vi "220117-VNA RP FLAT.vi"() -> ()   [LabVIEW 2021]
uses:
  b7fd31b3-4c8f-4ae8-a038-7c142e2eb182.vi
  <vilib>/Analysis/baseanly.llb/Mean (DBL).vi
  <vilib>/Utility/file.llb/Write Delimited Spreadsheet (DBL).vi
  <vilib>/Comparison/Equal/Equal Functor/Equal Functor.lvclass
  <vilib>/Analysis/NI_AALBase.lvlib
panel:
  in  "BTN CONNECT":bool
  in  "RP VNA SETTING":T1={"F start"=200000, "F stop"=2000500, "Sweep size"=1000, "Decimation"=5000, "F_corr"=0, "Ph_OUT1"=0, "Ph_OUT2"=0, "OUT_Lvl1"=32700, "OUT_Lvl2"=32700, "GPIO"=0}
  in  "Amplitude(1V)":dbl=0.3 format="%#_13g"
  out "RP CONNECT":bool
  in  "VOA Calibration cluster":cluster{"PUMP":dbl[], "PROBE":dbl[]}
  out "TRACK DATA REL NO SMOOTHING":dbl[][](array[numeric])
  out "TRACK DATA ABS NO SMOOTHING":dbl[][](array[numeric])
  in  "BTN SAVE TRACK":bool
  in  "BTN STOP TRACK":bool
  out "TRACK REPOSITERY":path
  out "TRACK DATA REL":dbl[][](array[numeric])
  out "TRACK DATA ABS":dbl[][](array[numeric])
  out "Track File List":path[](array[path])
  out "Track Repositery List":path[](array[path])
  out "CHANNEL CHOSEN":i32
  in  "TRACK-STOP":bool
  out "STATUS":string="STOP"
  out "track data":dbl[](array[numeric])=[495490.5081042979, 495481.56129759253, 495478.2328599854, 495479.84884744807, 495476.377462383, 495478.7819904735]
  out "Information tips":string
  in  "PANEL VNA":bool
  in  "PANEL TRACKING":bool
  in  "BTN STOP":bool
  in  "PANEL GENERAL SETTINGS":bool
  in  "PANEL TRACK SETTINGS":bool
  out "MAIN TAB":T2(tab)
  out "ACQ Indicator":bool
  in  "PUMP":dbl(slide)=100.0 min=0.0 max=100.0 step=0.1 scale=0.0..100.0
  in  "PROBE":dbl(slide)=100.0 min=0.0 max=100.0 step=0.1 scale=0.0..100.0
  in  "BTN RESET VNA":bool
  in  "SPAN":dbl=1900.0 format="%#5.1f"
  in  "STOP":dbl=2000.0 format="%#5.1f"
  in  "CENTER":dbl=1050.0 format="%#5.1f"
  in  "BTN SAVE VNA STG TO TRACK":bool
  in  "BTN AF VNA":bool
  out "MAGNITUDE/PHASE":cluster{cluster{dbl, dbl}[]}[](graph)
  in  "CHANNEL CHOICE VNA":T3(radio)
  in  "BTN Center to max":bool
  in  "BTN ZOOM-":bool
  in  "BTN ZOOM+":bool
  in  "START":dbl=200.0 format="%#5.1f"
  out "SPACING":dbl=1900.0 min=0.0 max=100.0 step=0.5 format="%#5.1f"
  in  "Points N°":i32=1000 min=600 max=5000 step=1 format="%#4.4g"
  in  "BTN LOOP VNA":bool
  in  "BTN RUN VNA":bool
  in  "Hide/Show track data channel":bool[](array[boolean])
  in  "BTN AUTOSAVE RAW DATA":bool=TRUE
  in  "COMMENTS":string
  in  "ASSAY NAME":string
  in  "DELAY AFTER SWITCH (s)":i32
  in  "N°POINTS TO DISPLAY":i32=200
  in  "DISPLAY OPTION":u16(ring) items=["Absolute frequency", "Relative frequency (ppm)"]
  in  "DELAY BETWEEN TRIG (s)":i32
  in  "AVERAGE/POINT":dbl=1.0
  out "LIVE TRACK":dbl[][](graph)
  out "CHANNELS IND TRACK":T3(radio)
  in  "BTN RUN TRACK":bool
  in  "TEMPORAL SMOOTHING":i32=15
  in  "BTN NEW TRACK":bool
  in  "BTN PAUSE TRACK":bool
  in  "CHANNELS PARAMETERS":T4(array[cluster])=[{"START 2"=200.0, "STOP 2"=2000.5, "CENTER 2"=1050.0, "SPAN 2"=1800.0, "CHANNEL TRACK ?"=FALSE, "PUMP"=100.0, "PROBE"=100.0, "Points N° 2"=1000, "SPACING 2"=100.0}, {"START 2"=200.0, "STOP 2"=2000.0, "CENTER 2"=1100.0, "SPAN 2"=1800.0, "CHANNEL TRACK ?"=FALSE, "PUMP"=100.0, "PROBE"=100.0, "Points N° 2"=1000, "SPACING 2"=1800.0}, {"START 2"=200.0, "STOP 2"=2000.0, "CENTER 2"=1100.0, "SPAN 2"=1800.0, "CHANNEL TRACK ?"=FALSE, "PUMP"=100.0, "PROBE"=100.0, "Points N° 2"=1000, "SPACING 2"=1800.0}, {"START 2"=200.0, "STOP 2"=2000.0, "CENTER 2"=1100.0, "SPAN 2"=1800.0, "CHANNEL TRACK ?"=FALSE, "PUMP"=100.0, "PROBE"=100.0, "Points N° 2"=1000, "SPACING 2"=1800.0}, {"START 2"=200.0, "STOP 2"=2000.0, "CENTER 2"=1100.0, "SPAN 2"=1800.0, "CHANNEL TRACK ?"=FALSE, "PUMP"=100.0, "PROBE"=100.0, "Points N° 2"=1000, "SPACING 2"=1800.0}, {"START 2"=200.0, "STOP 2"=2000.0, "CENTER 2"=1100.0, "SPAN 2"=1800.0, "CHANNEL TRACK ?"=FALSE, "PUMP"=100.0, "PROBE"=100.0, "Points N° 2"=1000, "SPACING 2"=1800.0}, {"START 2"=200.0, "STOP 2"=2000.0, "CENTER 2"=1100.0, "SPAN 2"=1800.0, "CHANNEL TRACK ?"=FALSE, "PUMP"=100.0, "PROBE"=100.0, "Points N° 2"=1000, "SPACING 2"=1800.0}, {"START 2"=200.0, "STOP 2"=2000.0, "CENTER 2"=1100.0, "SPAN 2"=1800.0, "CHANNEL TRACK ?"=FALSE, "PUMP"=100.0, "PROBE"=100.0, "Points N° 2"=1000, "SPACING 2"=1800.0}, {"START 2"=200.0, "STOP 2"=2000.0, "CENTER 2"=1100.0, "SPAN 2"=1800.0, "CHANNEL TRACK ?"=FALSE, "PUMP"=100.0, "PROBE"=100.0, "Points N° 2"=1000, "SPACING 2"=1800.0}, {"START 2"=200.0, "STOP 2"=2000.0, "CENTER 2"=1100.0, "SPAN 2"=1800.0, "CHANNEL TRACK ?"=FALSE, "PUMP"=100.0, "PROBE"=100.0, "Points N° 2"=1000, "SPACING 2"=1800.0}, {"START 2"=200.0, "STOP 2"=2000.0, "CENTER 2"=1100.0, "SPAN 2"=1800.0, "CHANNEL TRACK ?"=FALSE, "PUMP"=100.0, "PROBE"=100.0, "Points N° 2"=1000, "SPACING 2"=1800.0}, {"START 2"=200.0, "STOP 2"=2000.0, "CENTER 2"=1100.0, "SPAN 2"=1800.0, "CHANNEL TRACK ?"=FALSE, "PUMP"=100.0, "PROBE"=100.0, "Points N° 2"=1000, "SPACING 2"=1800.0}, {"START 2"=200.0, "STOP 2"=2000.0, "CENTER 2"=1100.0, "SPAN 2"=1800.0, "CHANNEL TRACK ?"=FALSE, "PUMP"=100.0, "PROBE"=100.0, "Points N° 2"=1000, "SPACING 2"=1800.0}, {"START 2"=200.0, "STOP 2"=2000.0, "CENTER 2"=1100.0, "SPAN 2"=1800.0, "CHANNEL TRACK ?"=FALSE, "PUMP"=100.0, "PROBE"=100.0, "Points N° 2"=1000, "SPACING 2"=1800.0}, {"START 2"=200.0, "STOP 2"=2000.0, "CENTER 2"=1100.0, "SPAN 2"=1800.0, "CHANNEL TRACK ?"=FALSE, "PUMP"=100.0, "PROBE"=100.0, "Points N° 2"=1000, "SPACING 2"=1800.0}, {"START 2"=200.0, "STOP 2"=2000.0, "CENTER 2"=1100.0, "SPAN 2"=1800.0, "CHANNEL TRACK ?"=FALSE, "PUMP"=100.0, "PROBE"=100.0, "Points N° 2"=1000, "SPACING 2"=1800.0}] {"SPACING 2" min=0.0 max=100.0 step=0.5; "Points N° 2" min=0 max=100 step=1; "PROBE" min=0.0 max=100.0 step=0.5; "PUMP" min=0.0 max=100.0 step=0.5}
  out "CHANNEL IND SETTINGS":T5(radio)
  in  "TRACK DATA PARAMETERS":cluster{"MAIN FOLDER":path}={"MAIN FOLDER"=path "C:/SensWay Data"}
  in  "SPECTRUM POST PROCESSING PARAMETERS":cluster{"N° SMOOTHING POINTS":i32}={"N° SMOOTHING POINTS"=50}
  in  "AUTOFOCUS PARAMETERS":cluster{"ITERATIONS":i32}={"ITERATIONS"=5}
  in  "CHANNELS":T6
  in  "NETWORK PARAMETERS":T7={"RP-IP 1"="192.168.0.3", "RP-IP 2"="192.168.0.4", "RP-MAC 1"="", "RP-MAC 2"=""}
  in  "VNA DATA CLUSTER":T8
  in  "TRACK DATA CLUSTER":cluster{"CHANNEL":dbl, "KPI 1 TRACK":ext[]}
  out "LOOP ACT":bool
  out "RAW Freq table":dbl[](array[numeric])=[200000.0, 201802.3023023023, 203604.6046046046, 205406.9069069069, 207209.20920920922, 209011.51151151152, 210813.81381381382, 212616.1161161161, 214418.4184184184, 216220.7207207207, 218023.02302302304, 219825.32532532534, 221627.62762762763, 223429.92992992993, 225232.23223223223, 227034.53453453453, 228836.83683683682, 230639.13913913915, 232441.44144144145, 234243.74374374375, 236046.04604604605, 237848.34834834834, 239650.65065065064, 241452.95295295294, 243255.25525525527, 245057.55755755756, 246859.85985985986, 248662.16216216216, 250464.46446446446, 252266.76676676676, 254069.06906906905, 255871.37137137138, 257673.67367367368, 259475.97597597598, 261278.27827827827, 263080.5805805806, 264882.8828828829, 266685.18518518517, 268487.4874874875, 270289.7897897898, 272092.0920920921, 273894.39439439436, 275696.6966966967, 277498.998998999, 279301.3013013013, 281103.6036036036, 282905.9059059059, 284708.2082082082, 286510.51051051053, 288312.8128128128, 290115.1151151151, 291917.4174174174, 293719.7197197197, 295522.02202202205, 297324.3243243243, 299126.6266266266, 300928.9289289289, 302731.23123123124, 304533.5335335335, 306335.83583583584, 308138.1381381381, 309940.44044044043, 311742.74274274276, 313545.04504504503, 315347.34734734736, 317149.6496496496, 318951.95195195195, 320754.2542542543, 322556.55655655655, 324358.8588588588, 326161.16116116114, 327963.4634634635, 329765.76576576574, 331568.06806806807, 333370.37037037034, 335172.67267267266, 336974.974974975, 338777.27727727726, 340579.5795795796, 342381.88188188185, 344184.1841841842, 345986.4864864865, 347788.7887887888, 349591.09109109105, 351393.3933933934, 353195.6956956957, 354997.997997998, 356800.3003003003, 358602.60260260256, 360404.9049049049, 362207.2072072072, 364009.50950950955, 365811.8118118118, 367614.1141141141, 369416.4164164164, 371218.71871871874, 373021.021021021, 374823.3233233233, 376625.6256256256, 378427.9279279279, 380230.23023023026, 382032.5325325325, 383834.8348348348, 385637.1371371371, 387439.43943943945, 389241.7417417418, 391044.04404404404, 392846.3463463463, 394648.64864864864, 396450.95095095097, 398253.25325325324, 400055.5555555555, 401857.85785785783, 403660.16016016016, 405462.4624624625, 407264.76476476475, 409067.067067067, 410869.36936936935, 412671.6716716717, 414473.973973974, 416276.2762762763, 418078.57857857854, 419880.88088088087, 421683.1831831832, 423485.48548548546, 425287.7877877878, 427090.09009009006, 428892.3923923924, 430694.6946946947, 432496.996996997, 434299.29929929925, 436101.6016016016, 437903.9039039039, 439706.20620620623, 441508.5085085085, 443310.81081081077, 445113.1131131131, 446915.4154154154, 448717.7177177177, 450520.02002002, 452322.3223223223, 454124.6246246246, 455926.92692692694, 457729.2292292292, 459531.5315315315, 461333.8338338338, 463136.13613613613, 464938.4384384384, 466740.74074074073, 468543.04304304306, 470345.3453453453, 472147.64764764765, 473949.9499499499, 475752.25225225225, 477554.5545545545, 479356.85685685684, 481159.1591591592, 482961.46146146144, 484763.76376376377, 486566.06606606604, 488368.36836836836, 490170.67067067063, 491972.97297297296, 493775.2752752753, 495577.57757757755, 497379.8798798799, 499182.18218218215, 500984.4844844845, 502786.78678678675, 504589.0890890891, 506391.3913913914, 508193.69369369367, 509995.995995996, 511798.29829829826, 513600.6006006006, 515402.90290290286, 517205.2052052052, 519007.5075075075, 520809.8098098098, 522612.1121121121, 524414.4144144144, 526216.7167167168, 528019.0190190191, 529821.3213213213, 531623.6236236236, 533425.9259259258, 535228.2282282282, 537030.5305305305, 538832.8328328328, 540635.1351351351, 542437.4374374375, 544239.7397397398, 546042.042042042, 547844.3443443443, 549646.6466466465, 551448.9489489489, 553251.2512512512, 555053.5535535535, 556855.8558558559, 558658.1581581582, 560460.4604604605, 562262.7627627627, 564065.065065065, 565867.3673673674, 567669.6696696696, 569471.9719719719, 571274.2742742742, 573076.5765765766, 574878.8788788789, 576681.1811811812, 578483.4834834835, 580285.7857857858, 582088.0880880881, 583890.3903903903, 585692.6926926926, 587494.994994995, 589297.2972972973, 591099.5995995996, 592901.9019019019, 594704.2042042043, 596506.5065065065, 598308.8088088088, 600111.111111111, 601913.4134134133, 603715.7157157157, 605518.018018018, 607320.3203203203, 609122.6226226226, 610924.924924925, 612727.2272272272, 614529.5295295295, 616331.8318318318, 618134.134134134, 619936.4364364364, 621738.7387387387, 623541.041041041, 625343.3433433434, 627145.6456456457, 628947.947947948, 630750.2502502502, 632552.5525525525, 634354.8548548548, 636157.1571571571, 637959.4594594594, 639761.7617617617, 641564.0640640641, 643366.3663663664, 645168.6686686687, 646970.9709709709, 648773.2732732733, 650575.5755755756, 652377.8778778778, 654180.1801801801, 655982.4824824824, 657784.7847847848, 659587.0870870871, 661389.3893893894, 663191.6916916918, 664993.993993994, 666796.2962962963, 668598.5985985985, 670400.9009009008, 672203.2032032032, 674005.5055055055, 675807.8078078078, 677610.1101101101, 679412.4124124125, 681214.7147147147, 683017.017017017, 684819.3193193192, 686621.6216216215, 688423.9239239239, 690226.2262262262, 692028.5285285285, 693830.8308308308, 695633.1331331332, 697435.4354354354, 699237.7377377377, 701040.04004004, 702842.3423423423, 704644.6446446446, 706446.9469469469, 708249.2492492492, 710051.5515515516, 711853.8538538539, 713656.1561561562, 715458.4584584584, 717260.7607607607, 719063.063063063, 720865.3653653653, 722667.6676676676, 724469.9699699699, 726272.2722722723, 728074.5745745746, 729876.8768768768, 731679.1791791791, 733481.4814814815, 735283.7837837838, 737086.0860860861, 738888.3883883883, 740690.6906906907, 742492.992992993, 744295.2952952953, 746097.5975975975, 747899.8998998998, 749702.2022022022, 751504.5045045045, 753306.8068068068, 755109.109109109, 756911.4114114114, 758713.7137137137, 760516.016016016, 762318.3183183183, 764120.6206206206, 765922.9229229229, 767725.2252252252, 769527.5275275275, 771329.8298298299, 773132.1321321321, 774934.4344344344, 776736.7367367367, 778539.039039039, 780341.3413413413, 782143.6436436436, 783945.9459459459, 785748.2482482482, 787550.5505505506, 789352.8528528528, 791155.1551551551, 792957.4574574574, 794759.7597597598, 796562.0620620621, 798364.3643643643, 800166.6666666666, 801968.968968969, 803771.2712712713, 805573.5735735735, 807375.8758758758, 809178.1781781781, 810980.4804804805, 812782.7827827828, 814585.085085085, 816387.3873873873, 818189.6896896897, 819991.991991992, 821794.2942942943, 823596.5965965965, 825398.8988988989, 827201.2012012012, 829003.5035035035, 830805.8058058057, 832608.108108108, 834410.4104104104, 836212.7127127127, 838015.015015015, 839817.3173173172, 841619.6196196196, 843421.9219219219, 845224.2242242242, 847026.5265265265, 848828.8288288288, 850631.1311311311, 852433.4334334334, 854235.7357357357, 856038.0380380381, 857840.3403403403, 859642.6426426426, 861444.9449449449, 863247.2472472473, 865049.5495495495, 866851.8518518518, 868654.1541541541, 870456.4564564564, 872258.7587587588, 874061.061061061, 875863.3633633633, 877665.6656656656, 879467.967967968, 881270.2702702703, 883072.5725725725, 884874.8748748748, 886677.1771771772, 888479.4794794795, 890281.7817817817, 892084.084084084, 893886.3863863864, 895688.6886886887, 897490.990990991, 899293.2932932932, 901095.5955955955, 902897.8978978979, 904700.2002002002, 906502.5025025025, 908304.8048048047, 910107.1071071071, 911909.4094094094, 913711.7117117117, 915514.0140140139, 917316.3163163163, 919118.6186186186, 920920.9209209209, 922723.2232232232, 924525.5255255254, 926327.8278278278, 928130.1301301301, 929932.4324324324, 931734.7347347348, 933537.037037037, 935339.3393393393, 937141.6416416416, 938943.943943944, 940746.2462462463, 942548.5485485485, 944350.8508508508, 946153.1531531531, 947955.4554554555, 949757.7577577577, 951560.06006006, 953362.3623623623, 955164.6646646647, 956966.966966967, 958769.2692692692, 960571.5715715715, 962373.8738738738, 964176.1761761762, 965978.4784784785, 967780.7807807807, 969583.083083083, 971385.3853853854, 973187.6876876877, 974989.9899899899, 976792.2922922922, 978594.5945945946, 980396.8968968969, 982199.1991991992, 984001.5015015014, 985803.8038038037, 987606.1061061061, 989408.4084084084, 991210.7107107107, 993013.0130130129, 994815.3153153153, 996617.6176176176, 998419.9199199199, 1000222.2222222221, 1002024.5245245245, 1003826.8268268268, 1005629.1291291291, 1007431.4314314314, 1009233.7337337337, 1011036.036036036, 1012838.3383383383, 1014640.6406406406, 1016442.942942943, 1018245.2452452452, 1020047.5475475475, 1021849.8498498498, 1023652.1521521521, 1025454.4544544544, 1027256.7567567567, 1029059.059059059, 1030861.3613613613, 1032663.6636636637, 1034465.9659659659, 1036268.2682682682, 1038070.5705705705, 1039872.8728728729, 1041675.1751751752, 1043477.4774774774, 1045279.7797797797, 1047082.082082082, 1048884.3843843844, 1050686.6866866867, 1052488.988988989, 1054291.2912912914, 1056093.5935935937, 1057895.895895896, 1059698.198198198, 1061500.5005005004, 1063302.8028028028, 1065105.105105105, 1066907.4074074074, 1068709.7097097095, 1070512.0120120118, 1072314.3143143142, 1074116.6166166165, 1075918.9189189188, 1077721.2212212211, 1079523.5235235235, 1081325.8258258258, 1083128.1281281281, 1084930.4304304305, 1086732.7327327328, 1088535.035035035, 1090337.3373373374, 1092139.6396396398, 1093941.9419419419, 1095744.2442442442, 1097546.5465465465, 1099348.8488488488, 1101151.1511511512, 1102953.4534534533, 1104755.7557557556, 1106558.058058058, 1108360.3603603602, 1110162.6626626626, 1111964.964964965, 1113767.2672672672, 1115569.5695695695, 1117371.8718718719, 1119174.1741741742, 1120976.4764764765, 1122778.7787787789, 1124581.0810810812, 1126383.3833833835, 1128185.6856856856, 1129987.987987988, 1131790.2902902903, 1133592.5925925926, 1135394.894894895, 1137197.197197197, 1138999.4994994993, 1140801.8018018017, 1142604.104104104, 1144406.4064064063, 1146208.7087087086, 1148011.011011011, 1149813.3133133133, 1151615.6156156156, 1153417.917917918, 1155220.2202202203, 1157022.5225225226, 1158824.824824825, 1160627.1271271273, 1162429.4294294294, 1164231.7317317317, 1166034.034034034, 1167836.3363363363, 1169638.6386386384, 1171440.9409409408, 1173243.243243243, 1175045.5455455454, 1176847.8478478477, 1178650.15015015, 1180452.4524524524, 1182254.7547547547, 1184057.057057057, 1185859.3593593594, 1187661.6616616617, 1189463.963963964, 1191266.2662662663, 1193068.5685685687, 1194870.8708708708, 1196673.173173173, 1198475.4754754754, 1200277.7777777778, 1202080.08008008, 1203882.3823823822, 1205684.6846846845, 1207486.9869869868, 1209289.2892892892, 1211091.5915915915, 1212893.8938938938, 1214696.1961961961, 1216498.4984984985, 1218300.8008008008, 1220103.103103103, 1221905.4054054054, 1223707.7077077078, 1225510.01001001, 1227312.3123123124, 1229114.6146146145, 1230916.9169169168, 1232719.2192192192, 1234521.5215215215, 1236323.8238238238, 1238126.126126126, 1239928.4284284282, 1241730.7307307306, 1243533.033033033, 1245335.3353353352, 1247137.6376376376, 1248939.9399399399, 1250742.2422422422, 1252544.5445445445, 1254346.8468468469, 1256149.1491491492, 1257951.4514514515, 1259753.7537537536, 1261556.056056056, 1263358.3583583583, 1265160.6606606606, 1266962.962962963, 1268765.2652652652, 1270567.5675675676, 1272369.86986987, 1274172.1721721722, 1275974.4744744743, 1277776.7767767766, 1279579.079079079, 1281381.3813813813, 1283183.6836836836, 1284985.985985986, 1286788.2882882883, 1288590.5905905906, 1290392.892892893, 1292195.195195195, 1293997.4974974974, 1295799.7997997997, 1297602.102102102, 1299404.4044044043, 1301206.7067067067, 1303009.009009009, 1304811.3113113113, 1306613.6136136136, 1308415.915915916, 1310218.218218218, 1312020.5205205204, 1313822.8228228227, 1315625.125125125, 1317427.4274274274, 1319229.7297297297, 1321032.032032032, 1322834.3343343344, 1324636.6366366367, 1326438.9389389388, 1328241.241241241, 1330043.5435435434, 1331845.8458458458, 1333648.148148148, 1335450.4504504504, 1337252.7527527527, 1339055.055055055, 1340857.3573573574, 1342659.6596596597, 1344461.9619619618, 1346264.2642642641, 1348066.5665665665, 1349868.8688688688, 1351671.1711711711, 1353473.4734734735, 1355275.7757757758, 1357078.078078078, 1358880.3803803804, 1360682.6826826825, 1362484.9849849849, 1364287.2872872872, 1366089.5895895895, 1367891.8918918918, 1369694.1941941942, 1371496.4964964965, 1373298.7987987988, 1375101.1011011011, 1376903.4034034032, 1378705.7057057056, 1380508.008008008, 1382310.3103103102, 1384112.6126126125, 1385914.9149149149, 1387717.2172172172, 1389519.5195195195, 1391321.8218218219, 1393124.1241241242, 1394926.4264264263, 1396728.7287287286, 1398531.031031031, 1400333.3333333333, 1402135.6356356356, 1403937.937937938, 1405740.2402402402, 1407542.5425425426, 1409344.844844845, 1411147.147147147, 1412949.4494494493, 1414751.7517517516, 1416554.054054054, 1418356.3563563563, 1420158.6586586586, 1421960.960960961, 1423763.2632632633, 1425565.5655655656, 1427367.867867868, 1429170.17017017, 1430972.4724724723, 1432774.7747747747, 1434577.077077077, 1436379.3793793793, 1438181.6816816817, 1439983.983983984, 1441786.2862862863, 1443588.5885885886, 1445390.8908908907, 1447193.193193193, 1448995.4954954954, 1450797.7977977977, 1452600.1001001, 1454402.4024024024, 1456204.7047047047, 1458007.007007007, 1459809.3093093093, 1461611.6116116114, 1463413.9139139138, 1465216.216216216, 1467018.5185185184, 1468820.8208208208, 1470623.123123123, 1472425.4254254254, 1474227.7277277277, 1476030.03003003, 1477832.3323323324, 1479634.6346346345, 1481436.9369369368, 1483239.2392392391, 1485041.5415415415, 1486843.8438438438, 1488646.146146146, 1490448.4484484484, 1492250.7507507508, 1494053.053053053, 1495855.3553553552, 1497657.6576576575, 1499459.9599599598, 1501262.2622622622, 1503064.5645645645, 1504866.8668668668, 1506669.1691691692, 1508471.4714714715, 1510273.7737737738, 1512076.0760760761, 1513878.3783783782, 1515680.6806806806, 1517482.9829829829, 1519285.2852852852, 1521087.5875875875, 1522889.8898898899, 1524692.1921921922, 1526494.4944944945, 1528296.7967967968, 1530099.099099099, 1531901.4014014013, 1533703.7037037036, 1535506.006006006, 1537308.3083083082, 1539110.6106106106, 1540912.912912913, 1542715.2152152152, 1544517.5175175176, 1546319.8198198196, 1548122.122122122, 1549924.4244244243, 1551726.7267267266, 1553529.029029029, 1555331.3313313313, 1557133.6336336336, 1558935.935935936, 1560738.2382382383, 1562540.5405405406, 1564342.8428428427, 1566145.145145145, 1567947.4474474473, 1569749.7497497497, 1571552.052052052, 1573354.3543543543, 1575156.6566566566, 1576958.958958959, 1578761.2612612613, 1580563.5635635634, 1582365.8658658657, 1584168.168168168, 1585970.4704704704, 1587772.7727727727, 1589575.075075075, 1591377.3773773774, 1593179.6796796797, 1594981.981981982, 1596784.2842842843, 1598586.5865865864, 1600388.8888888888, 1602191.191191191, 1603993.4934934934, 1605795.7957957957, 1607598.098098098, 1609400.4004004004, 1611202.7027027027, 1613005.005005005, 1614807.3073073071, 1616609.6096096095, 1618411.9119119118, 1620214.2142142141, 1622016.5165165165, 1623818.8188188188, 1625621.121121121, 1627423.4234234234, 1629225.7257257258, 1631028.0280280279, 1632830.3303303302, 1634632.6326326325, 1636434.9349349348, 1638237.2372372372, 1640039.5395395395, 1641841.8418418418, 1643644.1441441441, 1645446.4464464465, 1647248.7487487488, 1649051.051051051, 1650853.3533533532, 1652655.6556556555, 1654457.9579579579, 1656260.2602602602, 1658062.5625625625, 1659864.8648648649, 1661667.1671671672, 1663469.4694694695, 1665271.7717717716, 1667074.074074074, 1668876.3763763763, 1670678.6786786786, 1672480.980980981, 1674283.2832832832, 1676085.5855855856, 1677887.887887888, 1679690.1901901902, 1681492.4924924925, 1683294.7947947946, 1685097.097097097, 1686899.3993993993, 1688701.7017017016, 1690504.004004004, 1692306.3063063063, 1694108.6086086086, 1695910.910910911, 1697713.2132132133, 1699515.5155155153, 1701317.8178178177, 1703120.12012012, 1704922.4224224223, 1706724.7247247247, 1708527.027027027, 1710329.3293293293, 1712131.6316316316, 1713933.933933934, 1715736.236236236, 1717538.5385385384, 1719340.8408408407, 1721143.143143143, 1722945.4454454454, 1724747.7477477477, 1726550.05005005, 1728352.3523523523, 1730154.6546546547, 1731956.956956957, 1733759.259259259, 1735561.5615615614, 1737363.8638638637, 1739166.166166166, 1740968.4684684684, 1742770.7707707707, 1744573.073073073, 1746375.3753753754, 1748177.6776776777, 1749979.9799799798, 1751782.2822822821, 1753584.5845845845, 1755386.8868868868, 1757189.189189189, 1758991.4914914914, 1760793.7937937938, 1762596.096096096, 1764398.3983983984, 1766200.7007007005, 1768003.0030030028, 1769805.3053053052, 1771607.6076076075, 1773409.9099099098, 1775212.2122122122, 1777014.5145145145, 1778816.8168168168, 1780619.1191191191, 1782421.4214214215, 1784223.7237237236, 1786026.0260260259, 1787828.3283283282, 1789630.6306306305, 1791432.9329329329, 1793235.2352352352, 1795037.5375375375, 1796839.8398398398, 1798642.1421421422, 1800444.4444444443, 1802246.7467467466, 1804049.049049049, 1805851.3513513512, 1807653.6536536536, 1809455.955955956, 1811258.2582582582, 1813060.5605605606, 1814862.8628628629, 1816665.1651651652, 1818467.4674674673, 1820269.7697697696, 1822072.072072072, 1823874.3743743743, 1825676.6766766766, 1827478.978978979, 1829281.2812812813, 1831083.5835835836, 1832885.885885886, 1834688.188188188, 1836490.4904904903, 1838292.7927927927, 1840095.095095095, 1841897.3973973973, 1843699.6996996996, 1845502.002002002, 1847304.3043043043, 1849106.6066066066, 1850908.9089089087, 1852711.211211211, 1854513.5135135134, 1856315.8158158157, 1858118.118118118, 1859920.4204204204, 1861722.7227227227, 1863525.025025025, 1865327.3273273273, 1867129.6296296297, 1868931.9319319318, 1870734.234234234, 1872536.5365365364, 1874338.8388388387, 1876141.141141141, 1877943.4434434434, 1879745.7457457457, 1881548.048048048, 1883350.3503503504, 1885152.6526526525, 1886954.9549549548, 1888757.2572572571, 1890559.5595595594, 1892361.8618618618, 1894164.164164164, 1895966.4664664664, 1897768.7687687688, 1899571.071071071, 1901373.3733733734, 1903175.6756756755, 1904977.9779779778, 1906780.2802802802, 1908582.5825825825, 1910384.8848848848, 1912187.1871871871, 1913989.4894894895, 1915791.7917917918, 1917594.0940940941, 1919396.3963963962, 1921198.6986986985, 1923001.0010010009, 1924803.3033033032, 1926605.6056056055, 1928407.9079079079, 1930210.2102102102, 1932012.5125125125, 1933814.8148148148, 1935617.117117117, 1937419.4194194193, 1939221.7217217216, 1941024.024024024, 1942826.3263263262, 1944628.6286286286, 1946430.930930931, 1948233.2332332332, 1950035.5355355355, 1951837.8378378379, 1953640.14014014, 1955442.4424424423, 1957244.7447447446, 1959047.047047047, 1960849.3493493493, 1962651.6516516516, 1964453.953953954, 1966256.2562562563, 1968058.5585585586, 1969860.8608608607, 1971663.163163163, 1973465.4654654653, 1975267.7677677677, 1977070.07007007, 1978872.3723723723, 1980674.6746746746, 1982476.976976977, 1984279.2792792793, 1986081.5815815816, 1987883.8838838837, 1989686.186186186, 1991488.4884884884, 1993290.7907907907, 1995093.093093093, 1996895.3953953953, 1998697.6976976977, 2000500.0]
  in  "ENABLE INTERNAL MODULATION":bool=TRUE
  in  "VNA DATA CLUSTER TBL":T9(array[cluster])=[{"CHANNEL"=0.0, "FREQUENCY TABLE"=[0.0], "MAGNITUDE TABLE"=[0.0], "PHASE TABLE"=[0.0]}, {"CHANNEL"=1.0, "FREQUENCY TABLE"=[], "MAGNITUDE TABLE"=[], "PHASE TABLE"=[]}, {"CHANNEL"=2.0, "FREQUENCY TABLE"=[], "MAGNITUDE TABLE"=[], "PHASE TABLE"=[]}, {"CHANNEL"=3.0, "FREQUENCY TABLE"=[], "MAGNITUDE TABLE"=[], "PHASE TABLE"=[]}, {"CHANNEL"=4.0, "FREQUENCY TABLE"=[], "MAGNITUDE TABLE"=[], "PHASE TABLE"=[]}, {"CHANNEL"=5.0, "FREQUENCY TABLE"=[], "MAGNITUDE TABLE"=[], "PHASE TABLE"=[]}, {"CHANNEL"=6.0, "FREQUENCY TABLE"=[], "MAGNITUDE TABLE"=[], "PHASE TABLE"=[]}, {"CHANNEL"=7.0, "FREQUENCY TABLE"=[], "MAGNITUDE TABLE"=[], "PHASE TABLE"=[]}, {"CHANNEL"=8.0, "FREQUENCY TABLE"=[], "MAGNITUDE TABLE"=[], "PHASE TABLE"=[]}, {"CHANNEL"=9.0, "FREQUENCY TABLE"=[], "MAGNITUDE TABLE"=[], "PHASE TABLE"=[]}, {"CHANNEL"=10.0, "FREQUENCY TABLE"=[], "MAGNITUDE TABLE"=[], "PHASE TABLE"=[]}, {"CHANNEL"=11.0, "FREQUENCY TABLE"=[], "MAGNITUDE TABLE"=[], "PHASE TABLE"=[]}, {"CHANNEL"=12.0, "FREQUENCY TABLE"=[], "MAGNITUDE TABLE"=[], "PHASE TABLE"=[]}, {"CHANNEL"=13.0, "FREQUENCY TABLE"=[], "MAGNITUDE TABLE"=[], "PHASE TABLE"=[]}, {"CHANNEL"=14.0, "FREQUENCY TABLE"=[], "MAGNITUDE TABLE"=[], "PHASE TABLE"=[]}, {"CHANNEL"=15.0, "FREQUENCY TABLE"=[], "MAGNITUDE TABLE"=[], "PHASE TABLE"=[]}]
  in  "TRACK DATA CLUSTER TBL":cluster{"CHANNEL":dbl, "KPI 1 TRACK":ext[]}[](array[cluster])
  in  "VNA Settings cluster":T10={"START 2"=200.0, "STOP 2"=2000.5, "CENTER 2"=1050.0, "SPAN 2"=1901.0, "CHANNEL TRACK ?"=FALSE, "PUMP"=100.0, "PROBE"=100.0, "Points N° 2"=1000, "SPACING 2"=1901.0} {"SPACING 2" min=0.0 max=100.0 step=0.5; "Points N° 2" min=0 max=100 step=1; "PROBE" min=0.0 max=100.0 step=0.5; "PUMP" min=0.0 max=100.0 step=0.5}
  # "E"
  # "POINTS"
  # "SPACING"
  # "TRACK ?"
  # "START"
  # "STOP"
  # "CENTER"
  # "SPAN"
  # "PROBE"
  # "PUMP"
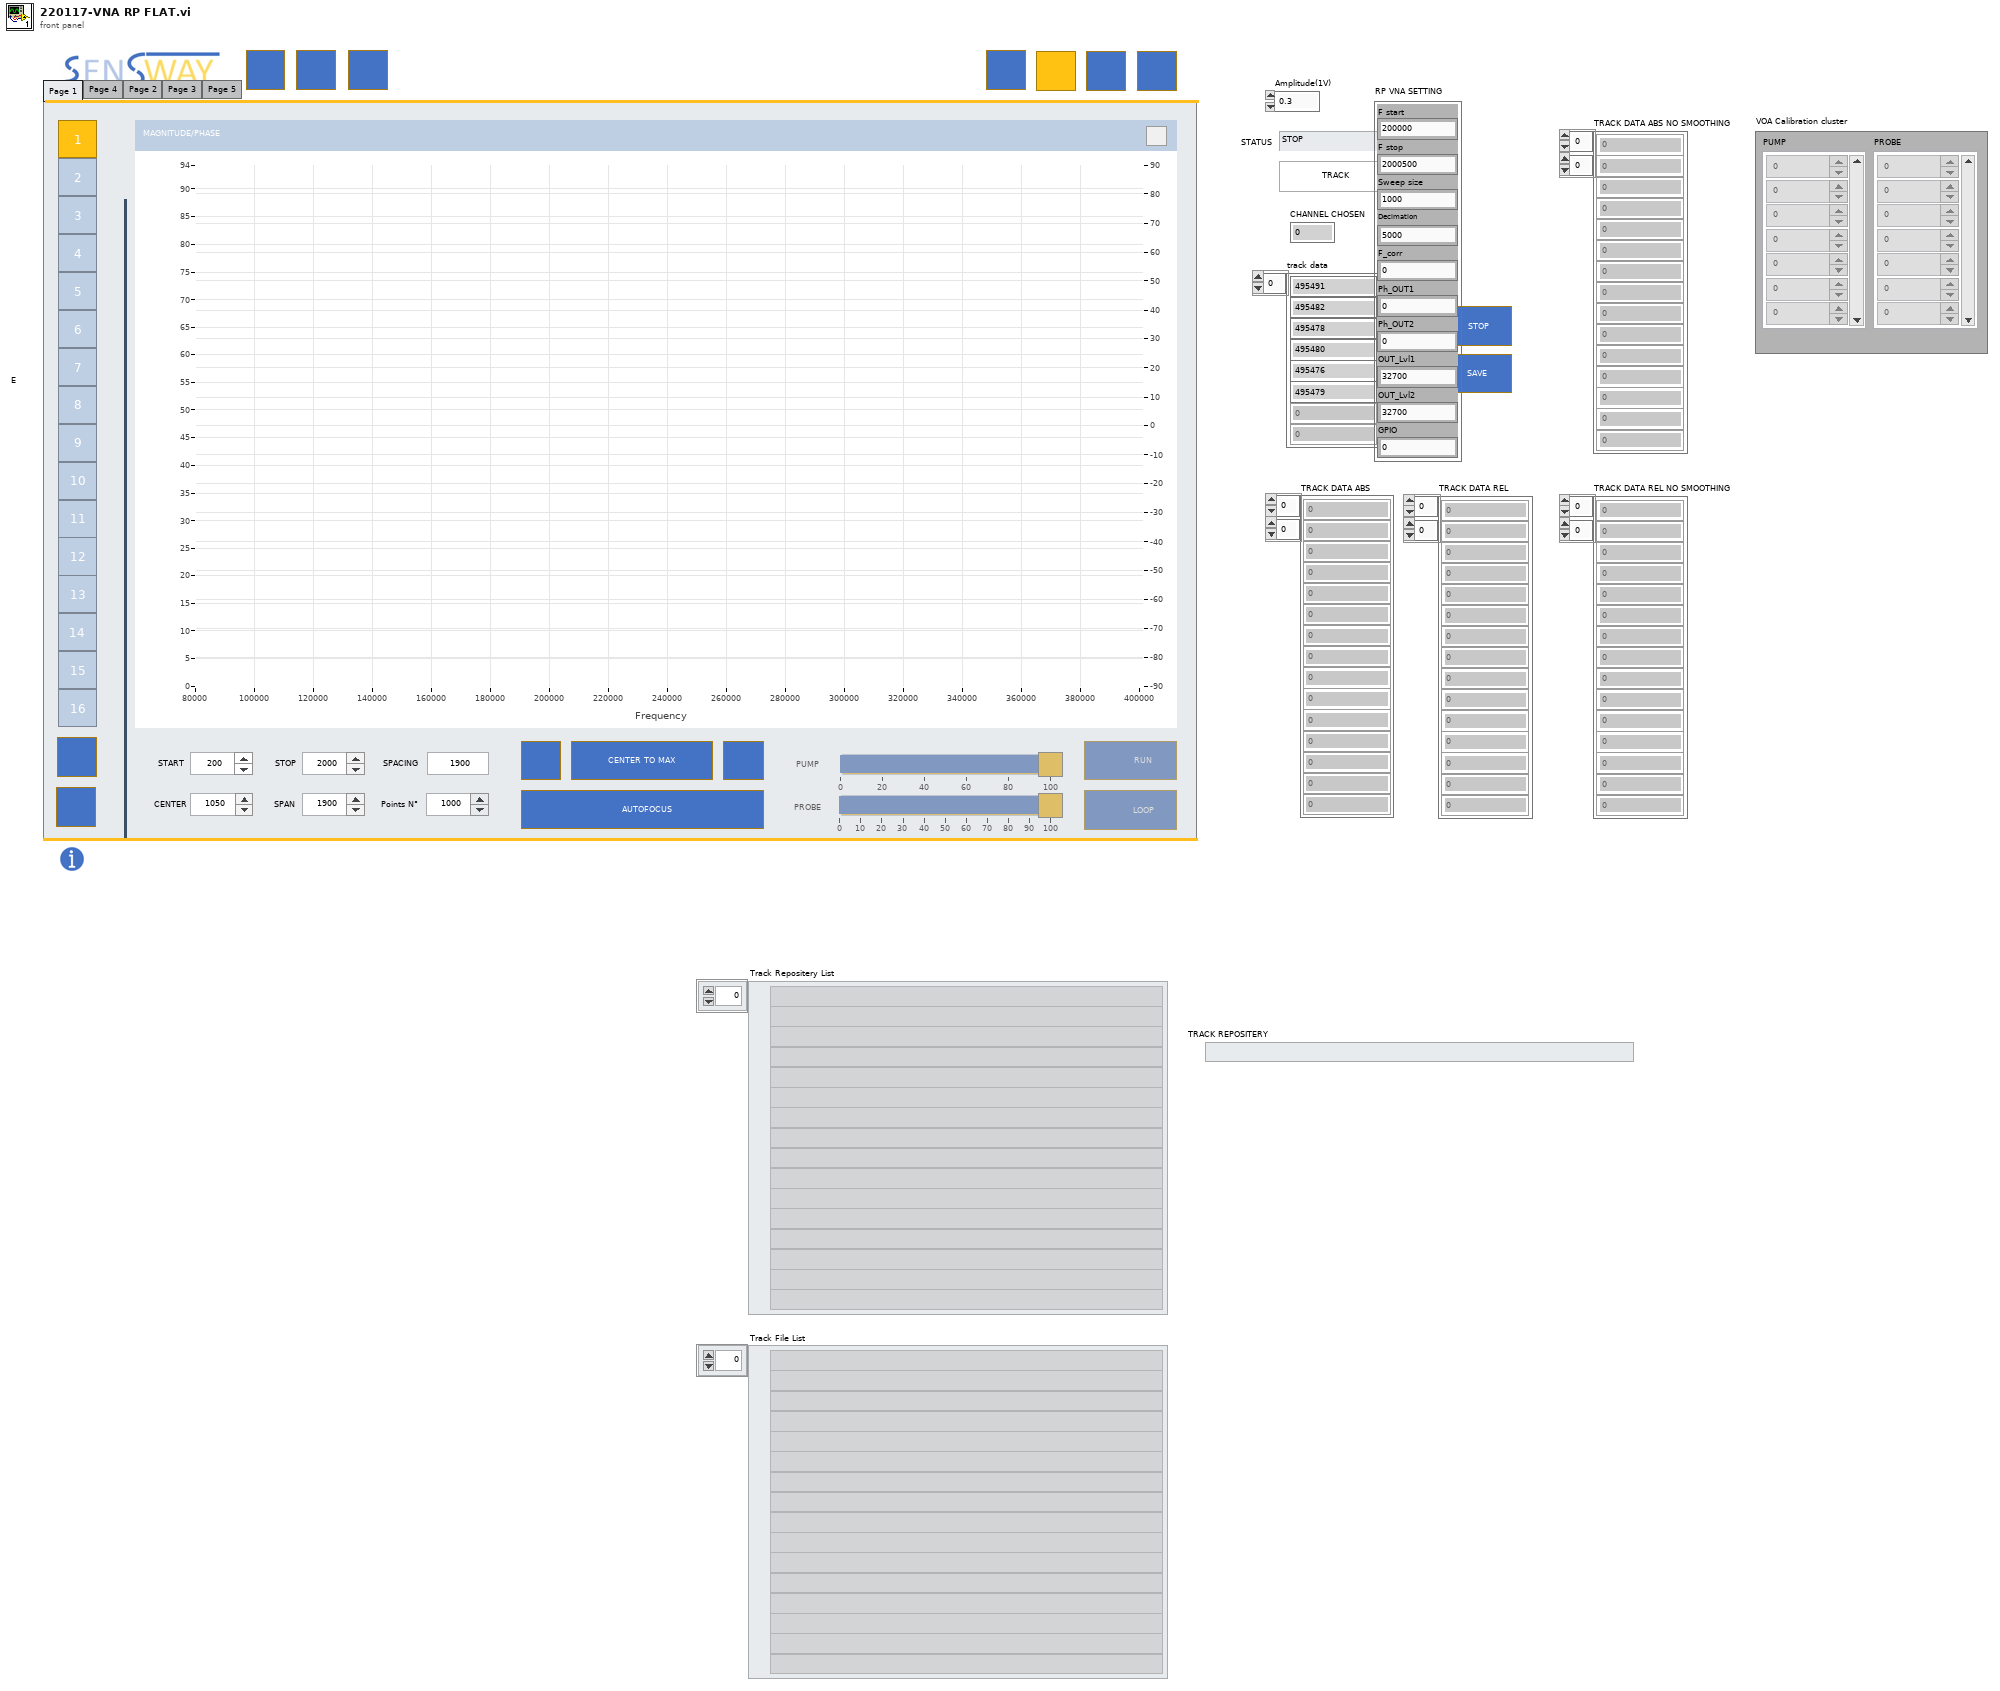
[diagram p1: front panel]
types:
  T1 = cluster{"F start":u32, "F stop":u32, "Sweep size":u32, "Decimation":u32, "F_corr":u32, "Ph_OUT1":u32, "Ph_OUT2":u32, "OUT_Lvl1":u32, "OUT_Lvl2":u32, "GPIO":u32}
  T2 = enum32{"Page 1", "Page 4", "Page 2", "Page 3", "Page 5"}
  T3 = enum32{"Button 1", "Button 2", "Button 3", "Sélection radio 4", "Sélection radio 5", "Sélection radio 6", "Sélection radio 7", "Sélection radio 8", "Sélection radio 9", "Sélection radio 10", "Sélection radio 11", "Sélection radio 12", "Sélection radio 13", "Sélection radio 14", "Sélection radio 15", "Sélection radio 16"}
  T4 = cluster{"START 2":dbl, "STOP 2":dbl, "CENTER 2":dbl, "SPAN 2":dbl, "CHANNEL TRACK ?":bool, "PUMP":dbl, "PROBE":dbl, "Points N° 2":i32, "SPACING 2":dbl}[]
  T5 = enum32{"No Selection", "Button 1", "Button 2", "Button 3", "Sélection radio 4", "Sélection radio 5", "Sélection radio 6", "Sélection radio 7", "Sélection radio 8", "Sélection radio 9", "Sélection radio 10", "Sélection radio 11", "Sélection radio 12", "Sélection radio 13", "Sélection radio 14", "Sélection radio 15", "Sélection radio 16"}
  T6 = cluster{"CHANNEL 1":bool, "CHANNEL 2":bool, "CHANNEL 3":bool, "CHANNEL 4":bool, "CHANNEL 5":bool, "CHANNEL 6":bool, "CHANNEL 7":bool, "CHANNEL 8":bool, "CHANNEL 9":bool, "CHANNEL 10":bool, "CHANNEL 11":bool, "CHANNEL 12":bool, "CHANNEL 13":bool, "CHANNEL 14":bool, "CHANNEL 15":bool, "CHANNEL 16":bool}
  T7 = cluster{"RP-IP 1":string, "RP-IP 2":string, "RP-MAC 1":string, "RP-MAC 2":string}
  T8 = cluster{"CHANNEL":dbl, "FREQUENCY TABLE":ext[], "MAGNITUDE TABLE":ext[], "PHASE TABLE":ext[]}
  T9 = cluster{"CHANNEL":dbl, "FREQUENCY TABLE":ext[], "MAGNITUDE TABLE":ext[], "PHASE TABLE":ext[]}[]
  T10 = cluster{"START 2":dbl, "STOP 2":dbl, "CENTER 2":dbl, "SPAN 2":dbl, "CHANNEL TRACK ?":bool, "PUMP":dbl, "PROBE":dbl, "Points N° 2":i32, "SPACING 2":dbl}
  T11 = enum16{"Freq start", "Freq stop", "Sweep size", "Decimation rate", "Freq corr", "Phase output 1", "Phase output 2", "Output level 1", "Output level 2", "GPIO", "SWEEP START"}
  T12 = enum8{"Enabled", "Disabled", "Disabled and Grayed Out"}
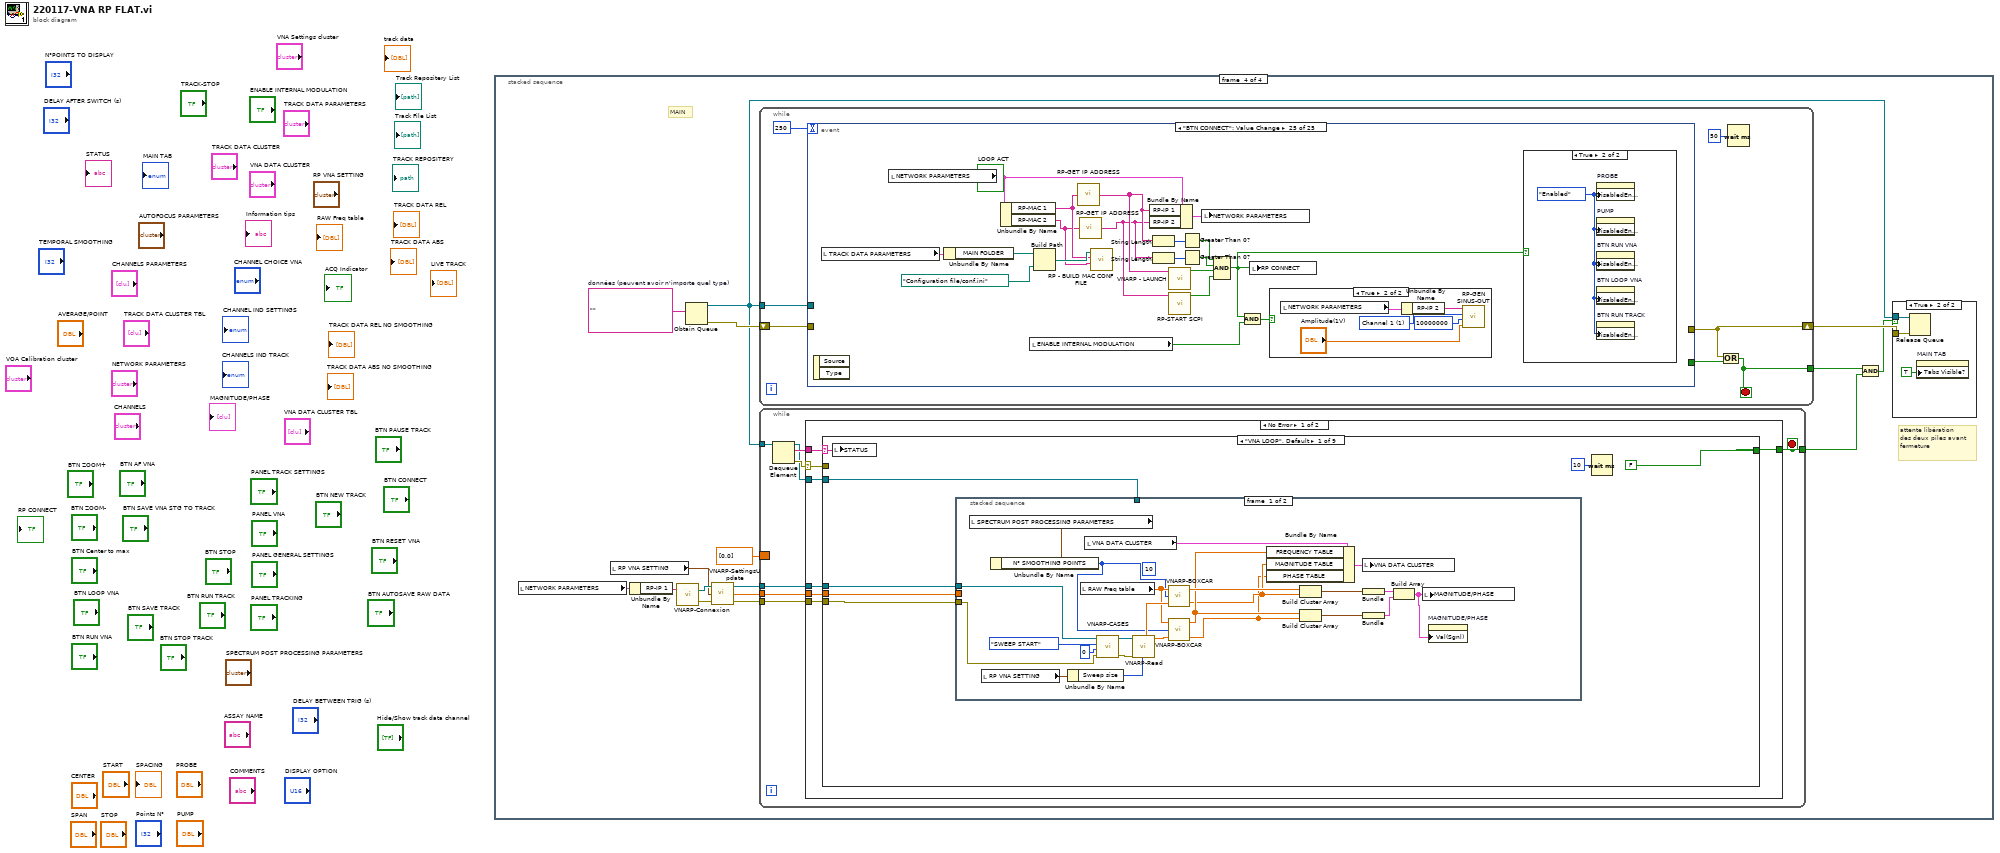
[diagram p0: block diagram]
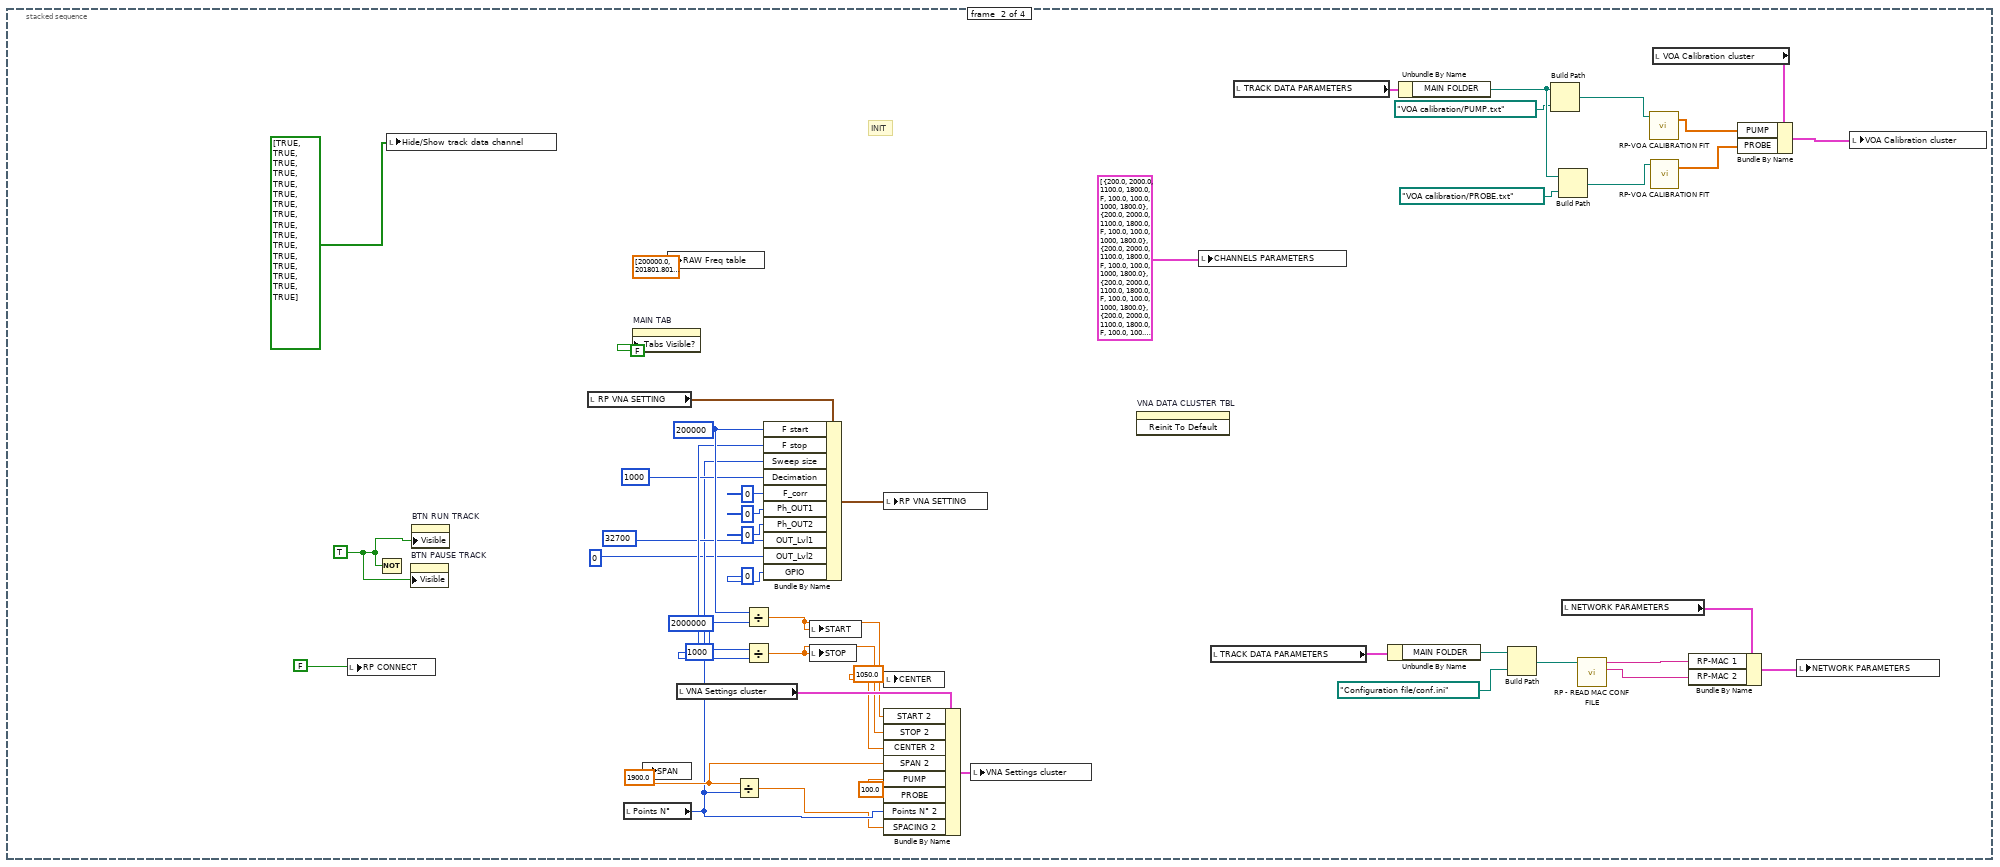
[diagram p3: hidden frame]
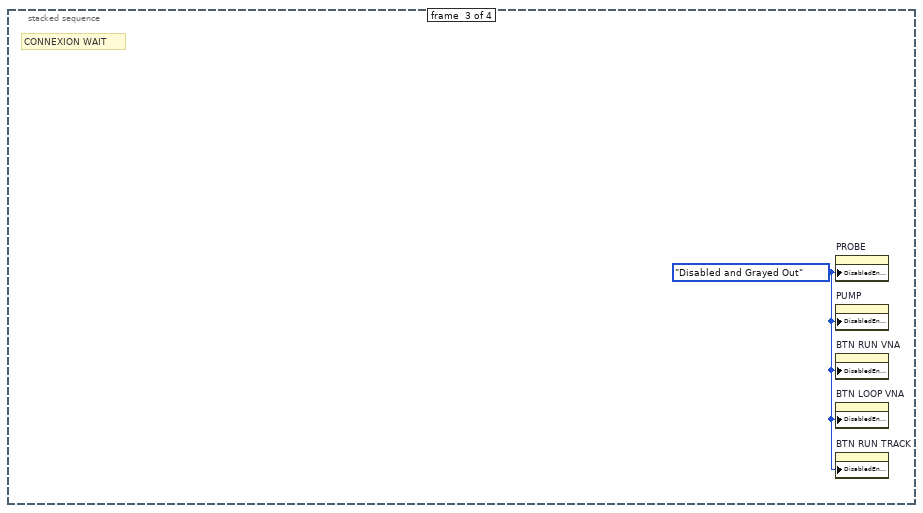
[diagram p4: hidden frame]
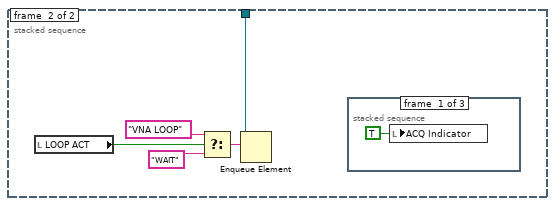
[diagram p6: hidden frame]
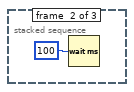
[diagram p7: hidden frame]
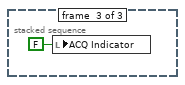
[diagram p8: hidden frame]
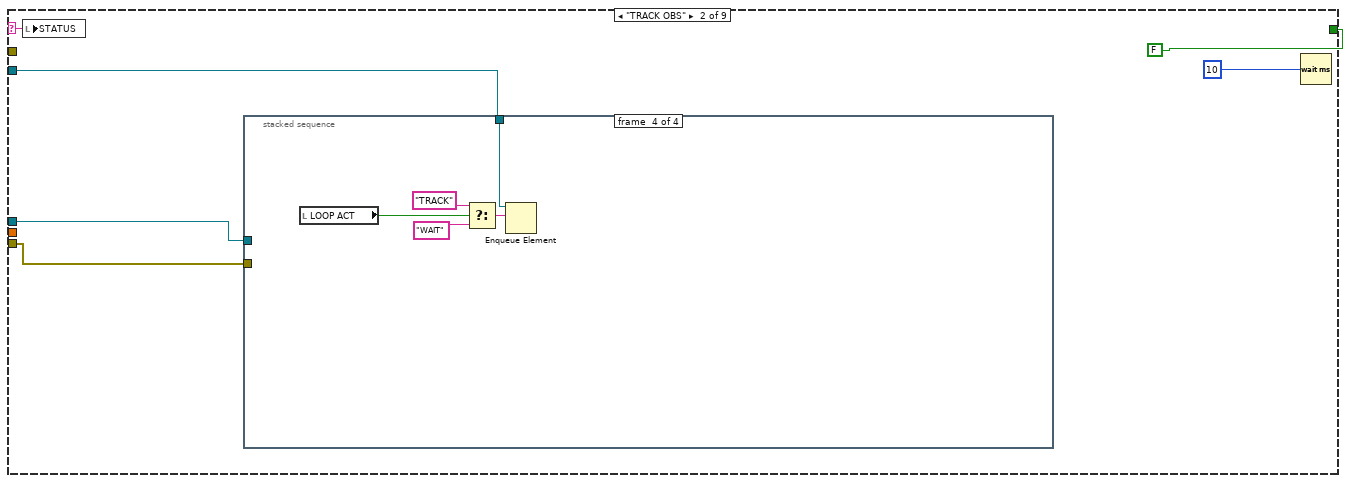
[diagram p9: hidden frame]
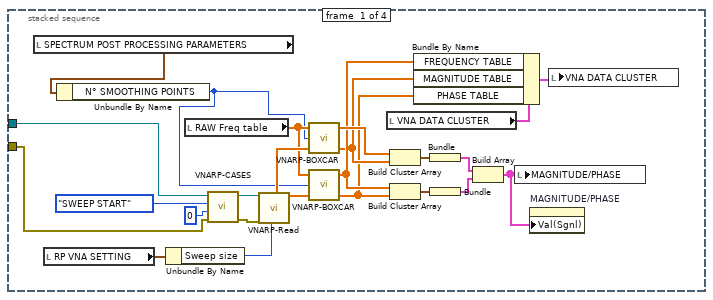
[diagram p10: hidden frame]
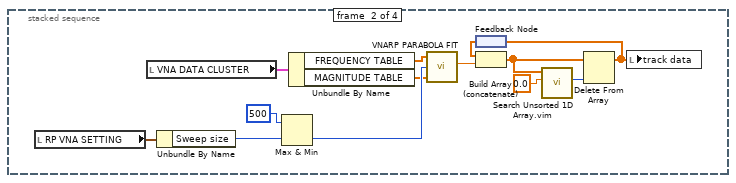
[diagram p11: hidden frame]
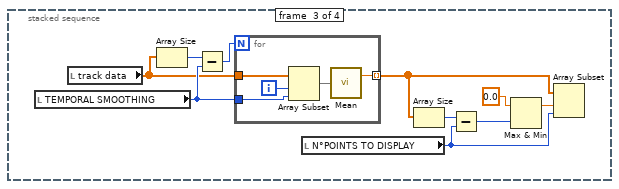
[diagram p12: hidden frame]
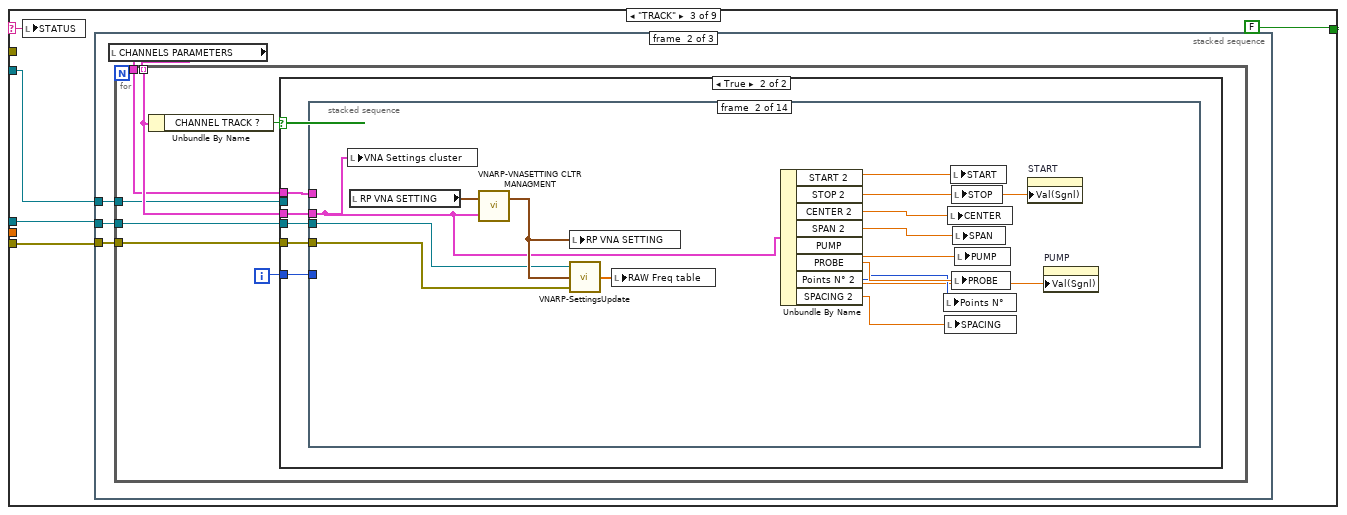
[diagram p13: hidden frame]
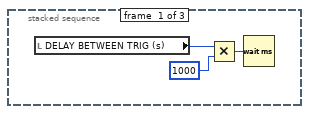
[diagram p14: hidden frame]
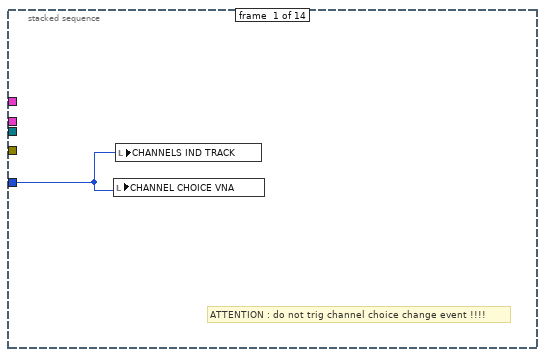
[diagram p16: hidden frame]
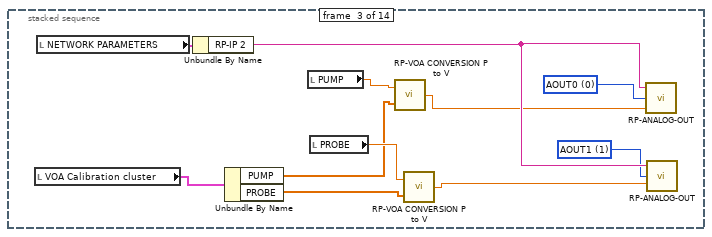
[diagram p17: hidden frame]
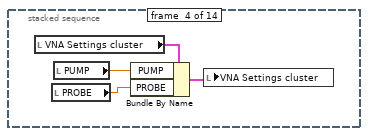
[diagram p18: hidden frame]
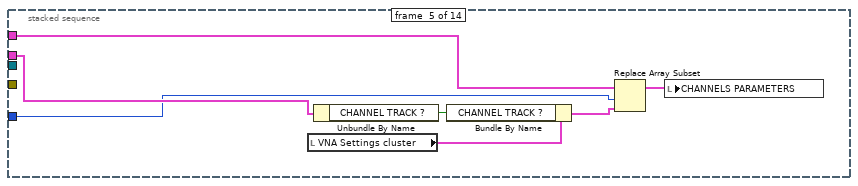
[diagram p19: hidden frame]
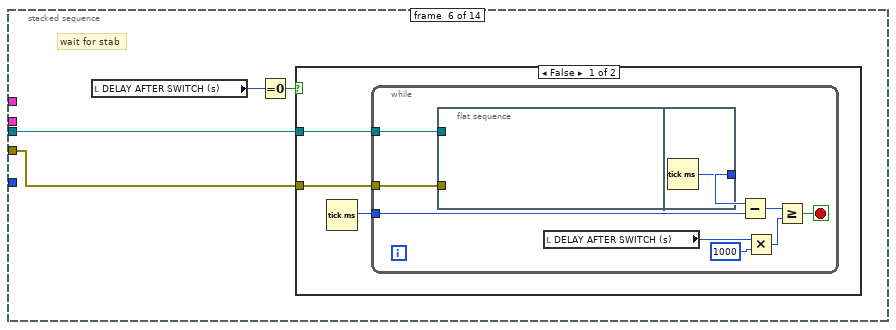
[diagram p20: hidden frame]
diagram:
  n1 = stacked-sequence {
    frame #0 {
    }
    frame #1 {
      w22 = TRUE ("x")
      w24 = 100.0 ("PUMP")
      w27 = 1900.0 ("Center")
      w28 = 1050.0 ("Center")
      w43 = u32 1000 ("Decimation")
      w41 = u32 2000000 ("Decimation")
      w42 = u32 200000 ("Decimation")
      # "INIT"
      n2 = local write "RP CONNECT"(FALSE) -> ()
      n3 = Not(x=w22) -> ()  [unwired: 1 out]
      n4 = local write "Hide/Show track data channel"(bool[] [TRUE, TRUE, TRUE, TRUE, TRUE, TRUE, TRUE, TRUE, TRUE, TRUE, TRUE, TRUE, TRUE, TRUE, TRUE, TRUE] ("Hide/Show track data channel")) -> ()
      n5 = property on="BTN PAUSE TRACK" class="Bool (strict)"("Visible"=w22) -> ()  [unwired: 2 in, 2 out]
      n6 = property on="BTN RUN TRACK" class="Bool (strict)"("Visible"=w22) -> ()  [unwired: 2 in, 2 out]
      n7 = local read "RP VNA SETTING"() -> (w45:T1)
      n8 = local read "Points N°"() -> (w26:i32)
      n9 = property on="MAIN TAB" class="TabCtl (strict)"("Tabs Visible?"=FALSE ("Onglets visibles ?")) -> ()  [unwired: 2 in, 2 out]
      n10 = local write "SPAN"(w27) -> ()
      n11 = local write "RAW Freq table"(dbl[] [200000.0, 201801.8018018018, 203603.6036036036, 205405.4054054054, 207207.20720720722, 209009.009009009, 210810.8108108108, 212612.6126126126, 214414.4144144144, 216216.2162162162, 218018.01801801802, 219819.81981981982, 221621.62162162163, 223423.42342342343, 225225.22522522524, 227027.02702702704, 228828.82882882882, 230630.63063063062, 232432.43243243243, 234234.23423423423, 236036.03603603604, 237837.83783783784, 239639.63963963964, 241441.44144144145, 243243.24324324325, 245045.04504504503, 246846.84684684683, 248648.64864864864, 250450.45045045044, 252252.25225225225, 254054.05405405405, 255855.85585585586, 257657.65765765766, 259459.45945945947, 261261.26126126124, 263063.0630630631, 264864.86486486485, 266666.6666666666, 268468.46846846846, 270270.2702702703, 272072.0720720721, 273873.87387387385, 275675.6756756757, 277477.47747747746, 279279.2792792793, 281081.08108108107, 282882.8828828829, 284684.6846846847, 286486.4864864865, 288288.2882882883, 290090.09009009006, 291891.8918918919, 293693.69369369367, 295495.4954954955, 297297.2972972973, 299099.0990990991, 300900.9009009009, 302702.7027027027, 304504.5045045045, 306306.3063063063, 308108.1081081081, 309909.90990990994, 311711.7117117117, 313513.5135135135, 315315.3153153153, 317117.1171171171, 318918.91891891893, 320720.7207207207, 322522.5225225225, 324324.3243243243, 326126.12612612615, 327927.9279279279, 329729.7297297297, 331531.53153153154, 333333.3333333333, 335135.13513513515, 336936.9369369369, 338738.7387387387, 340540.54054054053, 342342.34234234237, 344144.14414414414, 345945.9459459459, 347747.74774774775, 349549.5495495496, 351351.35135135136, 353153.15315315314, 354954.9549549549, 356756.75675675675, 358558.5585585586, 360360.36036036036, 362162.16216216213, 363963.96396396396, 365765.7657657658, 367567.5675675676, 369369.36936936935, 371171.1711711711, 372972.97297297296, 374774.7747747748, 376576.57657657657, 378378.37837837834, 380180.1801801802, 381981.981981982, 383783.7837837838, 385585.58558558556, 387387.38738738734, 389189.1891891892, 390990.990990991, 392792.7927927928, 394594.59459459456, 396396.3963963964, 398198.1981981982, 400000.0, 401801.8018018018, 403603.6036036036, 405405.4054054054, 407207.2072072072, 409009.009009009, 410810.81081081077, 412612.6126126126, 414414.41441441444, 416216.2162162162, 418018.018018018, 419819.8198198198, 421621.62162162166, 423423.42342342343, 425225.2252252252, 427027.027027027, 428828.8288288288, 430630.63063063065, 432432.4324324324, 434234.2342342342, 436036.03603603604, 437837.83783783787, 439639.63963963964, 441441.4414414414, 443243.2432432432, 445045.04504504503, 446846.84684684686, 448648.64864864864, 450450.4504504504, 452252.25225225225, 454054.0540540541, 455855.85585585586, 457657.65765765763, 459459.4594594594, 461261.26126126124, 463063.0630630631, 464864.86486486485, 466666.6666666666, 468468.46846846846, 470270.27027027024, 472072.0720720721, 473873.87387387385, 475675.6756756757, 477477.47747747746, 479279.2792792793, 481081.08108108107, 482882.8828828829, 484684.6846846847, 486486.48648648645, 488288.2882882883, 490090.09009009006, 491891.8918918919, 493693.69369369367, 495495.4954954955, 497297.2972972973, 499099.0990990991, 500900.9009009009, 502702.70270270266, 504504.5045045045, 506306.3063063063, 508108.1081081081, 509909.9099099099, 511711.7117117117, 513513.5135135135, 515315.3153153153, 517117.1171171171, 518918.91891891893, 520720.7207207207, 522522.5225225225, 524324.3243243243, 526126.1261261262, 527927.9279279279, 529729.7297297297, 531531.5315315316, 533333.3333333333, 535135.1351351351, 536936.9369369369, 538738.7387387387, 540540.5405405406, 542342.3423423423, 544144.1441441441, 545945.9459459459, 547747.7477477477, 549549.5495495496, 551351.3513513514, 553153.1531531531, 554954.9549549549, 556756.7567567567, 558558.5585585586, 560360.3603603604, 562162.1621621621, 563963.963963964, 565765.7657657657, 567567.5675675676, 569369.3693693693, 571171.1711711711, 572972.972972973, 574774.7747747747, 576576.5765765766, 578378.3783783783, 580180.1801801801, 581981.981981982, 583783.7837837838, 585585.5855855856, 587387.3873873875, 589189.1891891891, 590990.990990991, 592792.7927927928, 594594.5945945946, 596396.3963963964, 598198.1981981981, 600000.0, 601801.8018018018, 603603.6036036036, 605405.4054054054, 607207.2072072072, 609009.009009009, 610810.8108108108, 612612.6126126125, 614414.4144144144, 616216.2162162162, 618018.018018018, 619819.8198198199, 621621.6216216215, 623423.4234234234, 625225.2252252252, 627027.027027027, 628828.8288288289, 630630.6306306305, 632432.4324324324, 634234.2342342342, 636036.036036036, 637837.8378378379, 639639.6396396396, 641441.4414414414, 643243.2432432433, 645045.045045045, 646846.8468468469, 648648.6486486486, 650450.4504504504, 652252.2522522523, 654054.054054054, 655855.8558558559, 657657.6576576576, 659459.4594594594, 661261.2612612613, 663063.063063063, 664864.8648648649, 666666.6666666666, 668468.4684684684, 670270.2702702703, 672072.0720720721, 673873.8738738738, 675675.6756756757, 677477.4774774774, 679279.2792792793, 681081.0810810811, 682882.8828828828, 684684.6846846847, 686486.4864864864, 688288.2882882883, 690090.0900900901, 691891.8918918918, 693693.6936936937, 695495.4954954955, 697297.2972972973, 699099.099099099, 700900.9009009008, 702702.7027027027, 704504.5045045045, 706306.3063063063, 708108.1081081082, 709909.9099099098, 711711.7117117117, 713513.5135135135, 715315.3153153153, 717117.1171171172, 718918.9189189188, 720720.7207207207, 722522.5225225225, 724324.3243243243, 726126.1261261262, 727927.9279279279, 729729.7297297297, 731531.5315315315, 733333.3333333333, 735135.1351351351, 736936.9369369369, 738738.7387387387, 740540.5405405405, 742342.3423423424, 744144.1441441441, 745945.9459459459, 747747.7477477477, 749549.5495495496, 751351.3513513514, 753153.1531531531, 754954.9549549549, 756756.7567567567, 758558.5585585586, 760360.3603603604, 762162.1621621621, 763963.9639639639, 765765.7657657658, 767567.5675675676, 769369.3693693693, 771171.1711711711, 772972.9729729729, 774774.7747747748, 776576.5765765766, 778378.3783783783, 780180.1801801801, 781981.981981982, 783783.7837837838, 785585.5855855856, 787387.3873873873, 789189.1891891891, 790990.990990991, 792792.7927927928, 794594.5945945946, 796396.3963963963, 798198.1981981982, 800000.0, 801801.8018018018, 803603.6036036036, 805405.4054054053, 807207.2072072072, 809009.009009009, 810810.8108108108, 812612.6126126125, 814414.4144144144, 816216.2162162162, 818018.018018018, 819819.8198198198, 821621.6216216215, 823423.4234234234, 825225.2252252252, 827027.027027027, 828828.8288288288, 830630.6306306307, 832432.4324324324, 834234.2342342342, 836036.036036036, 837837.8378378379, 839639.6396396396, 841441.4414414414, 843243.2432432432, 845045.045045045, 846846.8468468469, 848648.6486486486, 850450.4504504504, 852252.2522522522, 854054.0540540541, 855855.8558558559, 857657.6576576576, 859459.4594594594, 861261.2612612612, 863063.0630630631, 864864.8648648649, 866666.6666666666, 868468.4684684684, 870270.2702702703, 872072.0720720721, 873873.8738738738, 875675.6756756756, 877477.4774774774, 879279.2792792793, 881081.0810810811, 882882.8828828828, 884684.6846846846, 886486.4864864865, 888288.2882882883, 890090.0900900901, 891891.8918918918, 893693.6936936936, 895495.4954954955, 897297.2972972973, 899099.099099099, 900900.9009009008, 902702.7027027027, 904504.5045045045, 906306.3063063063, 908108.108108108, 909909.9099099098, 911711.7117117117, 913513.5135135135, 915315.3153153153, 917117.117117117, 918918.9189189189, 920720.7207207207, 922522.5225225225, 924324.3243243243, 926126.1261261262, 927927.9279279279, 929729.7297297297, 931531.5315315315, 933333.3333333333, 935135.1351351351, 936936.9369369369, 938738.7387387387, 940540.5405405405, 942342.3423423424, 944144.1441441441, 945945.9459459459, 947747.7477477477, 949549.5495495495, 951351.3513513514, 953153.1531531531, 954954.9549549549, 956756.7567567567, 958558.5585585586, 960360.3603603604, 962162.1621621621, 963963.9639639639, 965765.7657657657, 967567.5675675676, 969369.3693693693, 971171.1711711711, 972972.9729729729, 974774.7747747748, 976576.5765765766, 978378.3783783783, 980180.1801801801, 981981.9819819819, 983783.7837837838, 985585.5855855856, 987387.3873873873, 989189.1891891891, 990990.990990991, 992792.7927927928, 994594.5945945946, 996396.3963963963, 998198.1981981982, 1000000.0, 1001801.8018018018, 1003603.6036036036, 1005405.4054054053, 1007207.2072072072, 1009009.009009009, 1010810.8108108108, 1012612.6126126125, 1014414.4144144144, 1016216.2162162162, 1018018.018018018, 1019819.8198198198, 1021621.6216216215, 1023423.4234234234, 1025225.2252252252, 1027027.027027027, 1028828.8288288288, 1030630.6306306307, 1032432.4324324324, 1034234.2342342342, 1036036.036036036, 1037837.8378378378, 1039639.6396396396, 1041441.4414414414, 1043243.2432432432, 1045045.045045045, 1046846.8468468469, 1048648.6486486485, 1050450.4504504504, 1052252.2522522523, 1054054.054054054, 1055855.8558558559, 1057657.6576576577, 1059459.4594594594, 1061261.261261261, 1063063.0630630632, 1064864.8648648649, 1066666.6666666665, 1068468.4684684684, 1070270.2702702703, 1072072.072072072, 1073873.8738738738, 1075675.6756756757, 1077477.4774774774, 1079279.2792792793, 1081081.0810810812, 1082882.8828828828, 1084684.6846846845, 1086486.4864864866, 1088288.2882882883, 1090090.09009009, 1091891.8918918918, 1093693.6936936937, 1095495.4954954954, 1097297.2972972973, 1099099.0990990992, 1100900.9009009008, 1102702.7027027027, 1104504.5045045046, 1106306.3063063063, 1108108.108108108, 1109909.9099099098, 1111711.7117117117, 1113513.5135135134, 1115315.3153153153, 1117117.1171171172, 1118918.9189189188, 1120720.7207207207, 1122522.5225225226, 1124324.3243243243, 1126126.126126126, 1127927.927927928, 1129729.7297297297, 1131531.5315315314, 1133333.3333333333, 1135135.1351351351, 1136936.9369369368, 1138738.7387387387, 1140540.5405405406, 1142342.3423423423, 1144144.1441441441, 1145945.945945946, 1147747.7477477477, 1149549.5495495494, 1151351.3513513515, 1153153.1531531531, 1154954.9549549548, 1156756.7567567567, 1158558.5585585586, 1160360.3603603602, 1162162.1621621621, 1163963.963963964, 1165765.7657657657, 1167567.5675675676, 1169369.3693693695, 1171171.1711711711, 1172972.9729729728, 1174774.774774775, 1176576.5765765766, 1178378.3783783782, 1180180.1801801801, 1181981.981981982, 1183783.7837837837, 1185585.5855855856, 1187387.3873873875, 1189189.189189189, 1190990.990990991, 1192792.792792793, 1194594.5945945946, 1196396.3963963962, 1198198.198198198, 1200000.0, 1201801.8018018017, 1203603.6036036036, 1205405.4054054054, 1207207.207207207, 1209009.009009009, 1210810.810810811, 1212612.6126126125, 1214414.4144144142, 1216216.2162162163, 1218018.018018018, 1219819.8198198196, 1221621.6216216215, 1223423.4234234234, 1225225.225225225, 1227027.027027027, 1228828.8288288289, 1230630.6306306305, 1232432.4324324324, 1234234.2342342343, 1236036.036036036, 1237837.8378378376, 1239639.6396396398, 1241441.4414414414, 1243243.243243243, 1245045.045045045, 1246846.8468468469, 1248648.6486486485, 1250450.4504504504, 1252252.2522522523, 1254054.054054054, 1255855.8558558559, 1257657.6576576575, 1259459.4594594594, 1261261.2612612613, 1263063.063063063, 1264864.8648648649, 1266666.6666666665, 1268468.4684684684, 1270270.2702702703, 1272072.072072072, 1273873.8738738738, 1275675.6756756757, 1277477.4774774774, 1279279.2792792793, 1281081.081081081, 1282882.8828828828, 1284684.6846846847, 1286486.4864864864, 1288288.2882882883, 1290090.09009009, 1291891.8918918918, 1293693.6936936937, 1295495.4954954954, 1297297.2972972973, 1299099.0990990992, 1300900.9009009008, 1302702.7027027027, 1304504.5045045044, 1306306.3063063063, 1308108.1081081082, 1309909.9099099098, 1311711.7117117117, 1313513.5135135134, 1315315.3153153153, 1317117.1171171172, 1318918.9189189188, 1320720.7207207207, 1322522.5225225224, 1324324.3243243243, 1326126.1261261262, 1327927.9279279278, 1329729.7297297297, 1331531.5315315316, 1333333.3333333333, 1335135.1351351351, 1336936.9369369368, 1338738.7387387387, 1340540.5405405406, 1342342.3423423423, 1344144.1441441441, 1345945.9459459458, 1347747.7477477477, 1349549.5495495496, 1351351.3513513512, 1353153.1531531531, 1354954.9549549548, 1356756.7567567567, 1358558.5585585586, 1360360.3603603602, 1362162.1621621621, 1363963.963963964, 1365765.7657657657, 1367567.5675675676, 1369369.3693693692, 1371171.1711711711, 1372972.972972973, 1374774.7747747747, 1376576.5765765766, 1378378.3783783782, 1380180.1801801801, 1381981.981981982, 1383783.7837837837, 1385585.5855855856, 1387387.3873873875, 1389189.189189189, 1390990.990990991, 1392792.7927927927, 1394594.5945945946, 1396396.3963963964, 1398198.198198198, 1400000.0, 1401801.8018018017, 1403603.6036036036, 1405405.4054054054, 1407207.207207207, 1409009.009009009, 1410810.8108108107, 1412612.6126126125, 1414414.4144144144, 1416216.216216216, 1418018.018018018, 1419819.8198198199, 1421621.6216216215, 1423423.4234234234, 1425225.225225225, 1427027.027027027, 1428828.8288288289, 1430630.6306306305, 1432432.4324324324, 1434234.234234234, 1436036.036036036, 1437837.8378378379, 1439639.6396396395, 1441441.4414414414, 1443243.243243243, 1445045.045045045, 1446846.8468468469, 1448648.6486486485, 1450450.4504504504, 1452252.2522522523, 1454054.054054054, 1455855.8558558559, 1457657.6576576575, 1459459.4594594594, 1461261.2612612613, 1463063.063063063, 1464864.8648648649, 1466666.6666666665, 1468468.4684684684, 1470270.2702702703, 1472072.072072072, 1473873.8738738738, 1475675.6756756757, 1477477.4774774774, 1479279.2792792793, 1481081.081081081, 1482882.8828828828, 1484684.6846846847, 1486486.4864864864, 1488288.2882882883, 1490090.09009009, 1491891.8918918918, 1493693.6936936937, 1495495.4954954954, 1497297.2972972973, 1499099.099099099, 1500900.9009009008, 1502702.7027027027, 1504504.5045045044, 1506306.3063063063, 1508108.1081081082, 1509909.9099099098, 1511711.7117117117, 1513513.5135135134, 1515315.3153153153, 1517117.1171171172, 1518918.9189189188, 1520720.7207207207, 1522522.5225225224, 1524324.3243243243, 1526126.1261261262, 1527927.9279279278, 1529729.7297297297, 1531531.5315315314, 1533333.3333333333, 1535135.1351351351, 1536936.9369369368, 1538738.7387387387, 1540540.5405405406, 1542342.3423423423, 1544144.1441441441, 1545945.9459459458, 1547747.7477477477, 1549549.5495495496, 1551351.3513513512, 1553153.1531531531, 1554954.9549549548, 1556756.7567567567, 1558558.5585585586, 1560360.3603603602, 1562162.1621621621, 1563963.963963964, 1565765.7657657657, 1567567.5675675676, 1569369.3693693692, 1571171.1711711711, 1572972.972972973, 1574774.7747747747, 1576576.5765765766, 1578378.3783783782, 1580180.1801801801, 1581981.981981982, 1583783.7837837837, 1585585.5855855856, 1587387.3873873872, 1589189.189189189, 1590990.990990991, 1592792.7927927927, 1594594.5945945946, 1596396.3963963964, 1598198.198198198, 1600000.0, 1601801.8018018017, 1603603.6036036036, 1605405.4054054054, 1607207.207207207, 1609009.009009009, 1610810.8108108107, 1612612.6126126125, 1614414.4144144144, 1616216.216216216, 1618018.018018018, 1619819.8198198196, 1621621.6216216215, 1623423.4234234234, 1625225.225225225, 1627027.027027027, 1628828.8288288289, 1630630.6306306305, 1632432.4324324324, 1634234.234234234, 1636036.036036036, 1637837.8378378379, 1639639.6396396395, 1641441.4414414414, 1643243.243243243, 1645045.045045045, 1646846.8468468469, 1648648.6486486485, 1650450.4504504504, 1652252.2522522523, 1654054.054054054, 1655855.8558558559, 1657657.6576576575, 1659459.4594594594, 1661261.2612612613, 1663063.063063063, 1664864.8648648649, 1666666.6666666665, 1668468.4684684684, 1670270.2702702703, 1672072.072072072, 1673873.8738738738, 1675675.6756756755, 1677477.4774774774, 1679279.2792792793, 1681081.081081081, 1682882.8828828828, 1684684.6846846847, 1686486.4864864864, 1688288.2882882883, 1690090.09009009, 1691891.8918918918, 1693693.6936936937, 1695495.4954954954, 1697297.2972972973, 1699099.099099099, 1700900.9009009008, 1702702.7027027027, 1704504.5045045044, 1706306.3063063063, 1708108.108108108, 1709909.9099099098, 1711711.7117117117, 1713513.5135135134, 1715315.3153153153, 1717117.1171171172, 1718918.9189189188, 1720720.7207207207, 1722522.5225225224, 1724324.3243243243, 1726126.1261261262, 1727927.9279279278, 1729729.7297297297, 1731531.5315315314, 1733333.3333333333, 1735135.1351351351, 1736936.9369369368, 1738738.7387387387, 1740540.5405405406, 1742342.3423423423, 1744144.1441441441, 1745945.9459459458, 1747747.7477477477, 1749549.5495495496, 1751351.3513513512, 1753153.1531531531, 1754954.9549549548, 1756756.7567567567, 1758558.5585585586, 1760360.3603603602, 1762162.1621621621, 1763963.9639639638, 1765765.7657657657, 1767567.5675675676, 1769369.3693693692, 1771171.1711711711, 1772972.972972973, 1774774.7747747747, 1776576.5765765766, 1778378.3783783782, 1780180.1801801801, 1781981.981981982, 1783783.7837837837, 1785585.5855855856, 1787387.3873873872, 1789189.189189189, 1790990.990990991, 1792792.7927927927, 1794594.5945945946, 1796396.3963963964, 1798198.198198198, 1800000.0, 1801801.8018018017, 1803603.6036036036, 1805405.4054054054, 1807207.207207207, 1809009.009009009, 1810810.8108108107, 1812612.6126126125, 1814414.4144144144, 1816216.216216216, 1818018.018018018, 1819819.8198198196, 1821621.6216216215, 1823423.4234234234, 1825225.225225225, 1827027.027027027, 1828828.8288288289, 1830630.6306306305, 1832432.4324324324, 1834234.234234234, 1836036.036036036, 1837837.8378378379, 1839639.6396396395, 1841441.4414414414, 1843243.243243243, 1845045.045045045, 1846846.8468468469, 1848648.6486486485, 1850450.4504504504, 1852252.252252252, 1854054.054054054, 1855855.8558558559, 1857657.6576576575, 1859459.4594594594, 1861261.2612612613, 1863063.063063063, 1864864.8648648649, 1866666.6666666665, 1868468.4684684684, 1870270.2702702703, 1872072.072072072, 1873873.8738738738, 1875675.6756756755, 1877477.4774774774, 1879279.2792792793, 1881081.081081081, 1882882.8828828828, 1884684.6846846847, 1886486.4864864864, 1888288.2882882883, 1890090.09009009, 1891891.8918918918, 1893693.6936936937, 1895495.4954954954, 1897297.2972972973, 1899099.099099099, 1900900.9009009008, 1902702.7027027027, 1904504.5045045044, 1906306.3063063063, 1908108.108108108, 1909909.9099099098, 1911711.7117117117, 1913513.5135135134, 1915315.3153153153, 1917117.1171171172, 1918918.9189189188, 1920720.7207207207, 1922522.5225225224, 1924324.3243243243, 1926126.1261261262, 1927927.9279279278, 1929729.7297297297, 1931531.5315315314, 1933333.3333333333, 1935135.1351351351, 1936936.9369369368, 1938738.7387387387, 1940540.5405405404, 1942342.3423423423, 1944144.1441441441, 1945945.9459459458, 1947747.7477477477, 1949549.5495495496, 1951351.3513513512, 1953153.1531531531, 1954954.9549549548, 1956756.7567567567, 1958558.5585585586, 1960360.3603603602, 1962162.1621621621, 1963963.9639639638, 1965765.7657657657, 1967567.5675675676, 1969369.3693693692, 1971171.1711711711, 1972972.972972973, 1974774.7747747747, 1976576.5765765766, 1978378.3783783782, 1980180.1801801801, 1981981.981981982, 1983783.7837837837, 1985585.5855855856, 1987387.3873873872, 1989189.189189189, 1990990.990990991, 1992792.7927927927, 1994594.5945945946, 1996396.3963963962, 1998198.198198198, 2000000.0] ("RAW Freq table")) -> ()
      n12 = local read "VNA Settings cluster"() -> (w32:T10)
      n13 = Divide(x=w27, y=w26) -> (x/y=w25:dbl)
      n14 = Divide(x=w42, y=w43) -> (x/y=w29:dbl)
      n15 = Divide(x=w41, y=w43) -> (x/y=w30:dbl)
      n16 = Bundle By Name(cluster=w45, "F start"=w42, "F stop"=w41, "Sweep size"=w26, "Decimation"=u32 1000, "F_corr"=u32 0, "Ph_OUT1"=u32 0, "Ph_OUT2"=u32 0 ("F_corr"), "OUT_Lvl1"=u32 32700 ("F_corr"), "OUT_Lvl2"=u32 0 ("F_corr"), "GPIO"=u32 0 ("F_corr")) -> (w44:T1)
      n17 = local write "START"(w29) -> ()
      n18 = local write "STOP"(w30) -> ()
      n19 = local write "RP VNA SETTING"(w44) -> ()
      n20 = local write "CENTER"(w28) -> ()
      n21 = Bundle By Name(cluster=w32, "START 2"=w29, "STOP 2"=w30, "CENTER 2"=w28, "SPAN 2"=w27, "PUMP"=w24, "PROBE"=w24, "Points N° 2"=w26, "SPACING 2"=w25) -> (w31:T10)
      n22 = local write "VNA Settings cluster"(w31) -> ()
      n23 = invoke on="VNA DATA CLUSTER TBL" class="Arr (strict)" method="Reinit To Default"() -> ()  [unwired: 3 in, 3 out]
      n24 = local write "CHANNELS PARAMETERS"(T4 [{"START 2"=200.0, "STOP 2"=2000.0, "CENTER 2"=1100.0, "SPAN 2"=1800.0, "CHANNEL TRACK ?"=FALSE, "PUMP"=100.0, "PROBE"=100.0, "Points N° 2"=1000, "SPACING 2"=1800.0}, {"START 2"=200.0, "STOP 2"=2000.0, "CENTER 2"=1100.0, "SPAN 2"=1800.0, "CHANNEL TRACK ?"=FALSE, "PUMP"=100.0, "PROBE"=100.0, "Points N° 2"=1000, "SPACING 2"=1800.0}, {"START 2"=200.0, "STOP 2"=2000.0, "CENTER 2"=1100.0, "SPAN 2"=1800.0, "CHANNEL TRACK ?"=FALSE, "PUMP"=100.0, "PROBE"=100.0, "Points N° 2"=1000, "SPACING 2"=1800.0}, {"START 2"=200.0, "STOP 2"=2000.0, "CENTER 2"=1100.0, "SPAN 2"=1800.0, "CHANNEL TRACK ?"=FALSE, "PUMP"=100.0, "PROBE"=100.0, "Points N° 2"=1000, "SPACING 2"=1800.0}, {"START 2"=200.0, "STOP 2"=2000.0, "CENTER 2"=1100.0, "SPAN 2"=1800.0, "CHANNEL TRACK ?"=FALSE, "PUMP"=100.0, "PROBE"=100.0, "Points N° 2"=1000, "SPACING 2"=1800.0}, {"START 2"=200.0, "STOP 2"=2000.0, "CENTER 2"=1100.0, "SPAN 2"=1800.0, "CHANNEL TRACK ?"=FALSE, "PUMP"=100.0, "PROBE"=100.0, "Points N° 2"=1000, "SPACING 2"=1800.0}, {"START 2"=200.0, "STOP 2"=2000.0, "CENTER 2"=1100.0, "SPAN 2"=1800.0, "CHANNEL TRACK ?"=FALSE, "PUMP"=100.0, "PROBE"=100.0, "Points N° 2"=1000, "SPACING 2"=1800.0}, {"START 2"=200.0, "STOP 2"=2000.0, "CENTER 2"=1100.0, "SPAN 2"=1800.0, "CHANNEL TRACK ?"=FALSE, "PUMP"=100.0, "PROBE"=100.0, "Points N° 2"=1000, "SPACING 2"=1800.0}, {"START 2"=200.0, "STOP 2"=2000.0, "CENTER 2"=1100.0, "SPAN 2"=1800.0, "CHANNEL TRACK ?"=FALSE, "PUMP"=100.0, "PROBE"=100.0, "Points N° 2"=1000, "SPACING 2"=1800.0}, {"START 2"=200.0, "STOP 2"=2000.0, "CENTER 2"=1100.0, "SPAN 2"=1800.0, "CHANNEL TRACK ?"=FALSE, "PUMP"=100.0, "PROBE"=100.0, "Points N° 2"=1000, "SPACING 2"=1800.0}, {"START 2"=200.0, "STOP 2"=2000.0, "CENTER 2"=1100.0, "SPAN 2"=1800.0, "CHANNEL TRACK ?"=FALSE, "PUMP"=100.0, "PROBE"=100.0, "Points N° 2"=1000, "SPACING 2"=1800.0}, {"START 2"=200.0, "STOP 2"=2000.0, "CENTER 2"=1100.0, "SPAN 2"=1800.0, "CHANNEL TRACK ?"=FALSE, "PUMP"=100.0, "PROBE"=100.0, "Points N° 2"=1000, "SPACING 2"=1800.0}, {"START 2"=200.0, "STOP 2"=2000.0, "CENTER 2"=1100.0, "SPAN 2"=1800.0, "CHANNEL TRACK ?"=FALSE, "PUMP"=100.0, "PROBE"=100.0, "Points N° 2"=1000, "SPACING 2"=1800.0}, {"START 2"=200.0, "STOP 2"=2000.0, "CENTER 2"=1100.0, "SPAN 2"=1800.0, "CHANNEL TRACK ?"=FALSE, "PUMP"=100.0, "PROBE"=100.0, "Points N° 2"=1000, "SPACING 2"=1800.0}, {"START 2"=200.0, "STOP 2"=2000.0, "CENTER 2"=1100.0, "SPAN 2"=1800.0, "CHANNEL TRACK ?"=FALSE, "PUMP"=100.0, "PROBE"=100.0, "Points N° 2"=1000, "SPACING 2"=1800.0}, {"START 2"=200.0, "STOP 2"=2000.0, "CENTER 2"=1100.0, "SPAN 2"=1800.0, "CHANNEL TRACK ?"=FALSE, "PUMP"=100.0, "PROBE"=100.0, "Points N° 2"=1000, "SPACING 2"=1800.0}] ("CHANNELS PARAMETERS")) -> ()
      n25 = local read "TRACK DATA PARAMETERS"() -> (w18:cluster{"MAIN FOLDER":path})
      n26 = local read "TRACK DATA PARAMETERS"() -> (w3:cluster{"MAIN FOLDER":path})
      n27 = Unbundle By Name(w18) -> ("MAIN FOLDER"=w17:path)
      n28 = Unbundle By Name(w3) -> ("MAIN FOLDER"=w4:path)
      n29 = Build Path(base path=w17, name or relative path=path "Configuration file/conf.ini") -> (appended path=w15:path)
      n30 = Build Path(base path=w4, name or relative path=path "VOA calibration/PUMP.txt") -> (appended path=w7:path)
      n31 = Build Path(base path=w4, name or relative path=path "VOA calibration/PROBE.txt") -> (appended path=w8:path)
      n32 = local read "NETWORK PARAMETERS"() -> (w14:T7)
      n33 = call "RP - READ MAC CONF FILE.vi"("Path"=w15) -> ("RP2 MAC"=w12:string, "RP1 MAC"=w13:string)  [unwired: 8 in, 1 out]
      n34 = call "RP-VOA CALIBRATION FIT.vi"("file path"=w7) -> ("Calibration array"=w9:dbl[])  [unwired: 2 in, 1 out]
      n35 = call "RP-VOA CALIBRATION FIT.vi"("file path"=w8) -> ("Calibration array"=w10:dbl[])  [unwired: 2 in, 1 out]
      n36 = local read "VOA Calibration cluster"() -> (w5:cluster{"PUMP":dbl[], "PROBE":dbl[]})
      n37 = Bundle By Name(cluster=w14, "RP-MAC 1"=w13, "RP-MAC 2"=w12) -> (w11:T7)
      n38 = Bundle By Name(cluster=w5, "PUMP"=w9, "PROBE"=w10) -> (w6:cluster{"PUMP":dbl[], "PROBE":dbl[]})
      n39 = local write "NETWORK PARAMETERS"(w11) -> ()
      n40 = local write "VOA Calibration cluster"(w6) -> ()
    }
    frame #2 {
      w46 = T12."Disabled and Grayed Out" ("Disabled")
      # "CONNEXION WAIT"
      n41 = property on="PROBE" class="Slide (strict)"("DisabledEnum"=w46) -> ()  [unwired: 2 in, 2 out]
      n42 = property on="PUMP" class="Slide (strict)"("DisabledEnum"=w46) -> ()  [unwired: 2 in, 2 out]
      n43 = property on="BTN RUN VNA" class="Bool (strict)"("DisabledEnum"=w46) -> ()  [unwired: 2 in, 2 out]
      n44 = property on="BTN LOOP VNA" class="Bool (strict)"("DisabledEnum"=w46) -> ()  [unwired: 2 in, 2 out]
      n45 = property on="BTN RUN TRACK" class="Bool (strict)"("DisabledEnum"=w46) -> ()  [unwired: 2 in, 2 out]
    }
    frame #3 {
      w60 = ""  # données (peuvent avoir n'importe quel type)
      # "attente libération des deux piles avant fermeture"
      # "MAIN"
      n46 = local read "NETWORK PARAMETERS"() -> (w49:T7)
      n47 = local read "RP VNA SETTING"() -> (w56:T1)
      n48 = Unbundle By Name(w49) -> ("RP-IP 1"=w48:string)
      n49 = call "VNARP-Connexion.vi"("IP RP"=w48) -> ("sortie d'erreur"=w58:errorcluster, "ID de connexion"=w57:refnum<k5>)  [unwired: 1 in]
      n50 = Obtain Queue(element data type=w60) -> (queue out=w59:refnum<queue>, error out=w62:errorcluster)  [unwired: 4 in, 1 out]
      n51 = call "VNARP-SettingsUpdate.vi"("Error IN"=w58, "RP VNA SETTINGS IN"=w56, "ID de connexion IN"=w57) -> ("Error OUT"=w53:errorcluster, "Freq table"=w54:dbl[], "ID de connexion OUT"=w55:refnum<k5>)
      n52 = while {
        shift-right: [w530] -> w61
        shift-left: w62 -> [w532]
        tunnel: w59 -> [w533]
        tunnel: [w528] -> w52
        stop <- w528 stop-if-true
        n53 = event shown="[24] \"BTN CONNECT\": Value Change" {
          selector: _ -> [_ _ _ _ _ _ _ _ _ _ _ _ _ _ _ _ _ _ _ _ _ _ _ _ _]
          dyn-events: _ -> [_ _ _ _ _ _ _ _ _ _ _ _ _ _ _ _ _ _ _ _ _ _ _ _ _]
          timeout: 250 -> [_ _ _ _ _ _ _ _ _ _ _ _ _ _ _ _ _ _ _ _ _ _ _ _ _]
          tunnel: w533 -> [w538 _ w545 w549 _ _ w566 _ w591 w613 w639 w665 w688 w700 w729 _ _ _ _ _ w742 _ w768 _ _]
          tunnel: w532 -> [w536 _ w544 w548 _ _ w565 _ w590 w612 w638 w667 w687 w699 w728 _ _ _ _ _ w741 _ w769 _ _]
          tunnel: [w535 _ w543 w547 _ _ w564 _ w589 w611 w636 w666 w686 w698 w730 _ _ _ _ _ w740 _ w767 _ _] -> w530
          tunnel: [_ _ _ _ _ _ _ _ _ _ _ _ _ _ w726 _ _ _ _ _ _ _ _ _ _] -> w531
          event "BTN LOOP VNA": Value Change {
            n54 = event-data() -> ("NewVal"=w534:bool)  [unwired: 1 in]
            n55 = local write "LOOP ACT"(w534) -> ()
            n56 = Enqueue Element(queue=w538, element="VNA LOOP", error in (no error)=w536) -> (error out=w535:errorcluster)  [unwired: 1 in, 2 out]
          }
          event "BTN SAVE VNA STG TO TRACK": Value Change {
            n57 = event-data() -> ()  [unwired: 1 in, 1 out]
            n58 = local read "CHANNELS PARAMETERS"() -> (w542:T4)
            n59 = local read "CHANNEL CHOICE VNA"() -> (w540:T3)
            n60 = local read "VNA Settings cluster"() -> (w539:T10)
            n61 = Replace Array Subset(array=w542, new element=w539, index=w540) -> (w541:T4)
            n62 = local write "CHANNELS PARAMETERS"(w541) -> ()
          }
          event "BTN RUN VNA": Value Change {
            n63 = event-data() -> ()  [unwired: 1 in, 2 out]
            n64 = Enqueue Element(queue=w545, element="RUN VNA", error in (no error)=w544) -> (error out=w543:errorcluster)  [unwired: 1 in, 2 out]
          }
          event "PUMP", "PROBE": Mouse Up {
            n65 = event-data() -> ()  [unwired: 1 in, 2 out]
            n66 = Enqueue Element(queue=w549, element="POWER UPDATE", error in (no error)=w548) -> (error out=w547:errorcluster)  [unwired: 1 in, 2 out]
          }
          event "Hide/Show track data channel": Value Change {
            # "TO TEST ON ALPHA"
            n67 = event-data() -> ()  [unwired: 1 in, 2 out]
            n68 = local read "Hide/Show track data channel"() -> (w551:bool[])
            n69 = for {
              tunnel: w551 -> [w552] mode=indexing
              i -> [w553]
              n70 = flat-sequence {
                tunnel: w553 -> [w554]
                tunnel: w552 -> [w555]
                frame #0 {
                  n71 = property on="LIVE TRACK" class="WFGraph (strict)"("Active Plot"=w554) -> ()  [unwired: 2 in, 2 out]
                }
                frame #1 {
                  n72 = property on="LIVE TRACK" class="WFGraph (strict)"("Plot.Visible?"=w555) -> ()  [unwired: 2 in, 2 out]
                }
              }
            }
          }
          event "MAGNITUDE/PHASE": Value Change {
            n73 = event-data() -> ()  [unwired: 1 in, 2 out]
            n74 = flat-sequence {
              frame #0 {
                n75 = property on="MAGNITUDE/PHASE" class="XYGraph (strict)"("ActYScl"=0 ("Active Y Scale")) -> ()  [unwired: 2 in, 2 out]
              }
              frame #1 {
                n76 = local read "VNA DATA CLUSTER"() -> (w560:T8)
                n77 = Unbundle By Name(w560) -> ("MAGNITUDE TABLE"=w561:ext[])
                n78 = Array Max & Min(array=w561) -> (max value=w562:ext)  [unwired: 3 out]
                n79 = Multiply(x=1.1, y=w562) -> (x*y=w558:ext)
                n80 = property on="MAGNITUDE/PHASE" class="XYGraph (strict)"("YScale.Maximum"=w558, "YScale.Minimum"=0.0) -> ()  [unwired: 2 in, 2 out]
              }
            }
          }
          event "CHANNEL CHOICE VNA": Value Change {
            n81 = event-data() -> ()  [unwired: 1 in, 2 out]
            n82 = Enqueue Element(queue=w566, element="CHANNEL CHANGE", error in (no error)=w565) -> (error out=w564:errorcluster)  [unwired: 1 in, 2 out]
            n83 = One Button Dialog(message="TRIGGERED !") -> ()  [unwired: 1 in, 1 out]
          }
          event "BTN NEW TRACK": Mouse Up {
            n84 = event-data() -> ()  [unwired: 1 in, 2 out]
            n85 = Two Button Dialog(message="Initiate a new tracking session ?") -> (T button?=w568:bool)  [unwired: 2 in]
            n86 = case shown="True" w568 {
              frame False {
              }
              frame True {
                n87 = stacked-sequence {
                  frame #0 {
                    # "LOCK ALL CONTROLS"
                  }
                  frame #1 {
                    n88 = local read "ASSAY NAME"() -> (w575:string)
                    n89 = local read "CHANNELS PARAMETERS"() -> (w576:T4)
                    n90 = local read "TRACK DATA PARAMETERS"() -> (w574:cluster{"MAIN FOLDER":path})
                    n91 = Unbundle By Name(w574) -> ("MAIN FOLDER"=w573:path)
                    n92 = call "RP-TRACKDataStructBuild.vi"("CHANNELS PARAMETERS"=w576, "Track session name"=w575, "SensWay track data path"=w573) -> ("TRACK REPOSITERY"=w572:path, "Track File List"=w571:path[], "Track Repositery List"=w570:path[])
                    n93 = local write "Track Repositery List"(w570) -> ()
                    n94 = local write "Track File List"(w571) -> ()
                    n95 = local write "TRACK REPOSITERY"(w572) -> ()
                  }
                  frame #2 {
                    n96 = local read "CHANNELS PARAMETERS"() -> (w578:T4)
                    n97 = for {
                      tunnel: w578 -> [w588] mode=indexing
                      border: cluster{"CHANNEL":dbl, "KPI 1 TRACK":ext[]}[] [] -> [_]
                      i -> [w584]
                      n98 = Unbundle By Name(w588) -> ("CHANNEL TRACK ?"=w579:bool)
                      n99 = Select(t=dbl[] [0.0], s=w579, f=dbl[] []) -> (s? t:f=w582:dbl[])
                      n100 = Bundle By Name(cluster=cluster{"CHANNEL":dbl, "KPI 1 TRACK":ext[]} {"CHANNEL"=0.0, "KPI 1 TRACK"=[0.0]} ("TRACK DATA CLUSTER"), "CHANNEL"=w584, "KPI 1 TRACK"=w582) -> (w583:cluster{"CHANNEL":dbl, "KPI 1 TRACK":ext[]})
                      n101 = feedback #1() -> (w586:cluster{"CHANNEL":dbl, "KPI 1 TRACK":ext[]}[])
                      n102 = Build Array (concatenate)(w586, w583) -> (w587:cluster{"CHANNEL":dbl, "KPI 1 TRACK":ext[]}[])
                      n103 = feedback-in #1(w587) -> ()
                      n104 = local write "TRACK DATA CLUSTER TBL"(w587) -> ()
                    }
                  }
                  frame #3 {
                  }
                }
              }
            }
          }
          event "START", "STOP": Value Change {
            n105 = event-data() -> ()  [unwired: 1 in, 1 out]
            n106 = stacked-sequence {
              frame #0 {
                n107 = local read "STOP"() -> (w597:dbl)
                n108 = local read "START"() -> (w596:dbl)
                n109 = Subtract(x=w597, y=w596) -> (x-y=w598:dbl)
                n110 = Add(x=w597, y=w596) -> (x+y=w595:dbl)
                n111 = local write "SPAN"(w598) -> ()
                n112 = Divide(x=w595, y=2.0) -> (x/y=w593:dbl)
                n113 = local write "CENTER"(w593) -> ()
              }
              frame #1 {
                n114 = local read "Points N°"() -> (w603:i32)
                n115 = local read "SPAN"() -> (w602:dbl)
                n116 = Divide(x=w602, y=w603) -> (x/y=w601:dbl)
                n117 = Multiply(x=w601, y=1000.0) -> (x*y=w600:dbl)
                n118 = local write "SPACING"(w600) -> ()
              }
              frame #2 {
                w604 = 1000
                n119 = local read "STOP"() -> (w606:dbl)
                n120 = local read "START"() -> (w608:dbl)
                n121 = Multiply(x=w608, y=w604) -> (x*y=w607:dbl)
                n122 = Multiply(x=w604, y=w606) -> (x*y=w605:dbl)
                n123 = local read "RP VNA SETTING"() -> (w610:T1)
                n124 = Bundle By Name(cluster=w610, "F start"=w607, "F stop"=w605) -> (w609:T1)
                n125 = local write "RP VNA SETTING"(w609) -> ()
              }
            }
            n126 = Enqueue Element(queue=w591, element="UPDATE", error in (no error)=w590) -> (error out=w589:errorcluster)  [unwired: 1 in, 2 out]
          }
          event "CENTER", "SPAN": Value Change {
            n127 = event-data() -> ()  [unwired: 1 in, 1 out]
            n128 = stacked-sequence {
              frame #0 {
                w616 = 100.0 ("y")
                n129 = local read "CENTER"() -> (w620:dbl)
                n130 = local read "SPAN"() -> (w622:dbl)
                n131 = Divide(x=w622, y=2.0) -> (x/y=w619:dbl)
                n132 = Subtract(x=w620, y=w619) -> (x-y=w617:dbl)
                n133 = Add(x=w620, y=w619) -> (x+y=w623:dbl)
                n134 = local write "STOP"(w623) -> ()
                n135 = Greater Or Equal?(x=w617, y=w616) -> (x >= y?=w618:bool)
                n136 = Select(t=w617, s=w618, f=w616) -> (s? t:f=w615:dbl)
                n137 = local write "START"(w615) -> ()
              }
              frame #1 {
                n138 = local read "Points N°"() -> (w628:i32)
                n139 = local read "SPAN"() -> (w627:dbl)
                n140 = Divide(x=w627, y=w628) -> (x/y=w626:dbl)
                n141 = Multiply(x=w626, y=1000.0) -> (x*y=w625:dbl)
                n142 = local write "SPACING"(w625) -> ()
              }
              frame #2 {
                w629 = 1000
                n143 = local read "STOP"() -> (w631:dbl)
                n144 = local read "START"() -> (w633:dbl)
                n145 = Multiply(x=w633, y=w629) -> (x*y=w632:dbl)
                n146 = Multiply(x=w629, y=w631) -> (x*y=w630:dbl)
                n147 = local read "RP VNA SETTING"() -> (w635:T1)
                n148 = Bundle By Name(cluster=w635, "F start"=w632, "F stop"=w630) -> (w634:T1)
                n149 = local write "RP VNA SETTING"(w634) -> ()
              }
            }
            n150 = Enqueue Element(queue=w613, element="UPDATE", error in (no error)=w612) -> (error out=w611:errorcluster)  [unwired: 1 in, 2 out]
          }
          event "BTN ZOOM+": Mouse Up; "BTN ZOOM+": Value Change {
            n151 = event-data() -> ()  [unwired: 1 in, 1 out]
            n152 = stacked-sequence {
              frame #0 {
                n153 = local read "SPAN"() -> (w642:dbl)
                n154 = Multiply(x=w642, y=0.8) -> (x*y=w640:dbl)
                n155 = local write "SPAN"(w640) -> ()
              }
              frame #1 {
                n156 = local read "Points N°"() -> (w647:i32)
                n157 = local read "SPAN"() -> (w646:dbl)
                n158 = Divide(x=w646, y=w647) -> (x/y=w645:dbl)
                n159 = Multiply(x=w645, y=1000.0) -> (x*y=w644:dbl)
                n160 = local write "SPACING"(w644) -> ()
              }
              frame #2 {
                w649 = 100.0 ("y")
                n161 = local read "SPAN"() -> (w652:dbl)
                n162 = local read "CENTER"() -> (w654:dbl)
                n163 = Divide(x=w652, y=2.0) -> (x/y=w653:dbl)
                n164 = Subtract(x=w654, y=w653) -> (x-y=w650:dbl)
                n165 = Add(x=w654, y=w653) -> (x+y=w656:dbl)
                n166 = local write "STOP"(w656) -> ()
                n167 = Greater Or Equal?(x=w650, y=w649) -> (x >= y?=w651:bool)
                n168 = Select(t=w650, s=w651, f=w649) -> (s? t:f=w648:dbl)
                n169 = local write "START"(w648) -> ()
              }
              frame #3 {
                w657 = 1000
                n170 = local read "STOP"() -> (w659:dbl)
                n171 = local read "START"() -> (w661:dbl)
                n172 = Multiply(x=w661, y=w657) -> (x*y=w660:dbl)
                n173 = Multiply(x=w657, y=w659) -> (x*y=w658:dbl)
                n174 = local read "RP VNA SETTING"() -> (w663:T1)
                n175 = Bundle By Name(cluster=w663, "F start"=w660, "F stop"=w658) -> (w662:T1)
                n176 = local write "RP VNA SETTING"(w662) -> ()
              }
            }
            n177 = Enqueue Element(queue=w639, element="UPDATE", error in (no error)=w638) -> (error out=w636:errorcluster)  [unwired: 1 in, 2 out]
          }
          event "BTN RESET VNA": Mouse Up {
            n178 = event-data() -> ()  [unwired: 1 in, 1 out]
            n179 = flat-sequence {
              tunnel: w665 -> [w669]
              tunnel: [w669] -> w664
              frame #0 {
                w678 = u32 1000 ("Decimation")
                w676 = u32 2000000 ("Decimation")
                w677 = u32 200000 ("Decimation")
                w671 = u32 32700 ("F_corr")
                n180 = local read "RP VNA SETTING"() -> (w681:T1)
                n181 = local read "Points N°"() -> (w679:i32)
                n182 = Bundle By Name(cluster=w681, "F start"=w677, "F stop"=w676, "Sweep size"=w679, "Decimation"=u32 5000, "F_corr"=u32 0, "Ph_OUT1"=u32 0, "Ph_OUT2"=u32 0 ("F_corr"), "OUT_Lvl1"=w671, "OUT_Lvl2"=w671, "GPIO"=u32 0 ("F_corr")) -> (w680:T1)
                n183 = local write "RP VNA SETTING"(w680) -> ()
                n184 = Divide(x=w676, y=w678) -> (x/y=w682:dbl)
                n185 = Divide(x=w677, y=w678) -> (x/y=w683:dbl)
                n186 = local write "CENTER"(1050.0 ("Center")) -> ()
                n187 = local write "SPAN"(1900.0 ("Center")) -> ()
                n188 = local write "START"(w683) -> ()
                n189 = local write "STOP"(w682) -> ()
              }
            }
            n190 = Enqueue Element(queue=w664, element="UPDATE", error in (no error)=w667) -> (error out=w666:errorcluster)  [unwired: 1 in, 2 out]
          }
          event "Points N°": Value Change {
            n191 = event-data() -> ()  [unwired: 1 in, 1 out]
            n192 = stacked-sequence {
              frame #0 {
                n193 = local read "Points N°"() -> (w694:i32)
                n194 = local read "SPAN"() -> (w693:dbl)
                n195 = Divide(x=w693, y=w694) -> (x/y=w692:dbl)
                n196 = Multiply(x=w692, y=1000.0) -> (x*y=w691:dbl)
                n197 = local write "SPACING"(w691) -> ()
              }
              frame #1 {
                n198 = local read "Points N°"() -> (w695:i32)
                n199 = local read "RP VNA SETTING"() -> (w697:T1)
                n200 = Bundle By Name(cluster=w697, "Sweep size"=w695) -> (w696:T1)
                n201 = local write "RP VNA SETTING"(w696) -> ()
              }
            }
            n202 = Enqueue Element(queue=w688, element="UPDATE", error in (no error)=w687) -> (error out=w686:errorcluster)  [unwired: 1 in, 2 out]
          }
          event "BTN ZOOM-": Mouse Up {
            n203 = event-data() -> ()  [unwired: 1 in, 1 out]
            n204 = stacked-sequence {
              frame #0 {
                n205 = local read "SPAN"() -> (w704:dbl)
                n206 = Multiply(x=w704, y=1.2) -> (x*y=w702:dbl)
                n207 = local write "SPAN"(w702) -> ()
              }
              frame #1 {
                n208 = local read "Points N°"() -> (w709:i32)
                n209 = local read "SPAN"() -> (w708:dbl)
                n210 = Divide(x=w708, y=w709) -> (x/y=w707:dbl)
                n211 = Multiply(x=w707, y=1000.0) -> (x*y=w706:dbl)
                n212 = local write "SPACING"(w706) -> ()
              }
              frame #2 {
                w712 = 100.0 ("y")
                n213 = local read "SPAN"() -> (w714:dbl)
                n214 = local read "CENTER"() -> (w717:dbl)
                n215 = Divide(x=w714, y=2.0) -> (x/y=w716:dbl)
                n216 = Subtract(x=w717, y=w716) -> (x-y=w710:dbl)
                n217 = Add(x=w717, y=w716) -> (x+y=w718:dbl)
                n218 = Greater Or Equal?(x=w710, y=w712) -> (x >= y?=w713:bool)
                n219 = Select(t=w710, s=w713, f=w712) -> (s? t:f=w711:dbl)
                n220 = local write "STOP"(w718) -> ()
                n221 = local write "START"(w711) -> ()
              }
              frame #3 {
                w719 = 1000
                n222 = local read "STOP"() -> (w721:dbl)
                n223 = local read "START"() -> (w723:dbl)
                n224 = Multiply(x=w723, y=w719) -> (x*y=w722:dbl)
                n225 = Multiply(x=w719, y=w721) -> (x*y=w720:dbl)
                n226 = local read "RP VNA SETTING"() -> (w725:T1)
                n227 = Bundle By Name(cluster=w725, "F start"=w722, "F stop"=w720) -> (w724:T1)
                n228 = local write "RP VNA SETTING"(w724) -> ()
              }
            }
            n229 = Enqueue Element(queue=w700, element="UPDATE", error in (no error)=w699) -> (error out=w698:errorcluster)  [unwired: 1 in, 2 out]
          }
          event "BTN STOP": Value Change {
            n230 = event-data() -> ()  [unwired: 1 in, 1 out]
            n231 = Two Button Dialog(message="Are you sure you want to exit ?") -> (T button?=w726:bool)  [unwired: 2 in]
            n232 = case shown="True" w726 {
              tunnel: [w731 w734] -> w730
              tunnel: w729 -> [_ w733]
              tunnel: w728 -> [w731 w732]
              frame False {
              }
              frame True {
                n233 = Enqueue Element(queue=w733, element="STOP", error in (no error)=w732) -> (error out=w734:errorcluster)  [unwired: 1 in, 2 out]
              }
            }
          }
          event "PANEL GENERAL SETTINGS": Value Change {
            n234 = event-data() -> ()  [unwired: 1 in, 2 out]
            n235 = local write "MAIN TAB"(enum32{"Page 1", "Page 4", "Page 2", "Page 3"}."Page 3" ("Tab Control")) -> ()
          }
          event Timeout {
            n236 = event-data() -> ()  [unwired: 1 in, 2 out]
          }
          event "PANEL TRACK SETTINGS": Value Change {
            n237 = event-data() -> ()  [unwired: 1 in, 2 out]
            n238 = local write "MAIN TAB"(enum32{"Page 1", "Page 4", "Page 2", "Page 3"}."Page 2" ("Tab Control")) -> ()
          }
          event "PANEL VNA": Value Change {
            n239 = event-data() -> ()  [unwired: 1 in, 2 out]
            n240 = local write "MAIN TAB"(enum32{"Page 1", "Page 4", "Page 2", "Page 3"}."Page 1" ("Tab Control")) -> ()
          }
          event "PANEL TRACKING": Value Change {
            n241 = event-data() -> ()  [unwired: 1 in, 2 out]
            n242 = local write "MAIN TAB"(enum32{"Page 1", "Page 4", "Page 2", "Page 3"}."Page 4" ("Tab Control")) -> ()
          }
          event "BTN Center to max": Mouse Up; "BTN Center to max": Value Change {
            n243 = event-data() -> ()  [unwired: 1 in, 2 out]
            n244 = stacked-sequence {
              frame #0 {
                # "ATTENTION ! CONFUSION  freq table"
                n245 = local read "VNA DATA CLUSTER"() -> (w747:T8)
                n246 = Unbundle By Name(w747) -> ("FREQUENCY TABLE"=w746:ext[], "MAGNITUDE TABLE"=w745:ext[])
                n247 = Array Max & Min(array=w745) -> (max index (indices)=w750:i32)  [unwired: 3 out]
                n248 = Index Array(array=w746, index=w750) -> (element=w749:ext)
                n249 = Divide(x=w749, y=1000.0) -> (x/y=w744:ext)
                n250 = local write "CENTER"(w744) -> ()
                n251 = property on="CENTER" class="DigNum (strict)"("Val(Sgnl)"=w744) -> ()  [unwired: 2 in, 2 out]
              }
              frame #1 {
                w753 = 1000
                n252 = local read "START"() -> (w751:dbl)
                n253 = local read "STOP"() -> (w752:dbl)
                n254 = Multiply(x=w751, y=w753) -> (x*y=w755:dbl)
                n255 = Multiply(x=w753, y=w752) -> (x*y=w754:dbl)
                n256 = local read "RP VNA SETTING"() -> (w757:T1)
                n257 = Bundle By Name(cluster=w757, "F start"=w755, "F stop"=w754) -> (w756:T1)
                n258 = local write "RP VNA SETTING"(w756) -> ()
              }
            }
            n259 = Enqueue Element(queue=w742, element="UPDATE", error in (no error)=w741) -> (error out=w740:errorcluster)  [unwired: 1 in, 2 out]
          }
          event "BTN AF VNA": Mouse Up {
            n260 = event-data() -> ()  [unwired: 1 in, 2 out]
            n261 = local read "AUTOFOCUS PARAMETERS"() -> (w759:cluster{"ITERATIONS":i32})
            n262 = Unbundle By Name(w759) -> ("ITERATIONS"=w758:i32)
            n263 = for {
              N: w758 -> [_]
              tunnel: [w762] -> w760
              n264 = flat-sequence {
                tunnel: [w763] -> w762
                frame #0 {
                  w763 = FALSE ("Valeur (Signalisation)")
                  n265 = property on="BTN Center to max" class="Bool (strict)"("Val(Sgnl)"=w763) -> ()  [unwired: 2 in, 2 out]
                }
                frame #1 {
                  n266 = property on="BTN ZOOM+" class="Bool (strict)"("Val(Sgnl)"=FALSE ("Valeur (Signalisation)")) -> ()  [unwired: 2 in, 2 out]
                }
              }
              n267 = Wait (ms)(milliseconds to wait=u32 250 ("attente (ms)")) -> ()  [unwired: 1 out]
            }
            n268 = property on="BTN Center to max" class="Bool (strict)"("Val(Sgnl)"=w760) -> ()  [unwired: 2 in, 2 out]
          }
          event "BTN RUN TRACK": Value Change {
            w765 = TRUE ("x")
            n269 = event-data() -> ()  [unwired: 1 in, 2 out]
            n270 = Not(x=w765) -> (.not. x?=w766:bool)
            n271 = local write "LOOP ACT"(w765) -> ()
            n272 = property on="BTN PAUSE TRACK" class="Bool (strict)"("Visible"=w765) -> ()  [unwired: 2 in, 2 out]
            n273 = Enqueue Element(queue=w768, element="TRACK", error in (no error)=w769) -> (error out=w767:errorcluster)  [unwired: 1 in, 2 out]
            n274 = property on="BTN RUN TRACK" class="Bool (strict)"("Visible"=w766) -> ()  [unwired: 2 in, 2 out]
          }
          event "BTN PAUSE TRACK": Mouse Up {
            w771 = FALSE ("x")
            n275 = event-data() -> ()  [unwired: 1 in, 2 out]
            n276 = Not(x=w771) -> (.not. x?=w772:bool)
            n277 = local write "LOOP ACT"(w771) -> ()
            n278 = property on="BTN PAUSE TRACK" class="Bool (strict)"("Visible"=w771) -> ()  [unwired: 2 in, 2 out]
            n279 = property on="BTN RUN TRACK" class="Bool (strict)"("Visible"=w772) -> ()  [unwired: 2 in, 2 out]
          }
          event "BTN CONNECT": Value Change {
            n280 = event-data() -> ()  [unwired: 1 in, 2 out]
            n281 = local read "TRACK DATA PARAMETERS"() -> (w781:cluster{"MAIN FOLDER":path})
            n282 = local read "NETWORK PARAMETERS"() -> (w782:T7)
            n283 = Unbundle By Name(w781) -> ("MAIN FOLDER"=w780:path)
            n284 = Unbundle By Name(w782) -> ("RP-MAC 1"=w778:string, "RP-MAC 2"=w777:string)
            n285 = local read "ENABLE INTERNAL MODULATION"() -> (w774:bool)
            n286 = Build Path(base path=w780, name or relative path=path "Configuration file/conf.ini") -> (appended path=w779:path)
            n287 = call "RP-GET IP ADDRESS.vi"("MAC address"=w778) -> ("IP address"=w787:string)
            n288 = call "RP-GET IP ADDRESS.vi"("MAC address"=w777) -> ("IP address"=w784:string)
            n289 = call "RP - BUILD MAC CONF FILE.vi"("RP2 MAC"=w777, "RP1 MAC"=w778, "Path"=w779) -> ()  [unwired: 8 in, 1 out]
            n290 = Bundle By Name(cluster=w782, "RP-IP 1"=w787, "RP-IP 2"=w784) -> (w791:T7)
            n291 = String Length(string=w787) -> (length=w789:i32)
            n292 = String Length(string=w784) -> (length=w790:i32)
            n293 = call "VNARP - LAUNCH.vi"("RP IP"=w787) -> ("VNA launched ?"=w788:bool)  [unwired: 10 in]
            n294 = call "RP-START SCPI.vi"("RP IP"=w784) -> ("SCPI launched ?"=w783:bool)  [unwired: 10 in]
            n295 = Greater Than 0?(x=w789) -> (x > 0?=w786:bool)
            n296 = Greater Than 0?(x=w790) -> (x > 0?=w785:bool)
            n297 = local write "NETWORK PARAMETERS"(w791) -> ()
            n298 = Compound Arithmetic op=AND(w786, w785, w788, w783) -> (w773:bool)
            n299 = And(x=w773, y=w774) -> (x .and. y?=w775:bool)
            n300 = local write "RP CONNECT"(w773) -> ()
            n301 = case shown="True" w775 {
              frame False {
              }
              frame True {
                w795 = u16 1 items=["Channel 1"=1, "Channel 2"=2] ("Channel (1|2)")
                n302 = local read "NETWORK PARAMETERS"() -> (w794:T7)
                n303 = Unbundle By Name(w794) -> ("RP-IP 2"=w793:string)
                n304 = call "RP-GEN SINUS-OUT.vi"("Amplitude(1V)"="Amplitude(1V)", "Frequency (Hz)"=10000000, "Channel (1|2)"=w795, "IP address"=w793) -> ()  [unwired: 1 out]
              }
            }
            n305 = case shown="True" w773 {
              frame False {
              }
              frame True {
                w792 = T12."Enabled" ("Disabled")
                n306 = property on="PROBE" class="Slide (strict)"("DisabledEnum"=w792) -> ()  [unwired: 2 in, 2 out]
                n307 = property on="PUMP" class="Slide (strict)"("DisabledEnum"=w792) -> ()  [unwired: 2 in, 2 out]
                n308 = property on="BTN RUN VNA" class="Bool (strict)"("DisabledEnum"=w792) -> ()  [unwired: 2 in, 2 out]
                n309 = property on="BTN LOOP VNA" class="Bool (strict)"("DisabledEnum"=w792) -> ()  [unwired: 2 in, 2 out]
                n310 = property on="BTN RUN TRACK" class="Bool (strict)"("DisabledEnum"=w792) -> ()  [unwired: 2 in, 2 out]
              }
            }
          }
        }
        n311 = Or(x=w530, y=w531) -> (x .or. y?=w528:bool)
        n312 = Wait (ms)(milliseconds to wait=u32 50 ("attente (ms)")) -> ()  [unwired: 1 out]
      }
      n313 = while {
        tunnel: w59 -> [w71]
        tunnel: w55 -> [w69]
        tunnel: w54 -> [w68]
        tunnel: w53 -> [w67]
        tunnel: [w66] -> w51
        border: dbl[] [0.0] -> [_]
        stop <- w66 stop-if-true
        n314 = Dequeue Element(queue=w71) -> (queue out=w70:refnum<queue>, element=w72:string, error out=w73:errorcluster)  [unwired: 2 in, 1 out]
        n315 = case shown="No Error" w73 {
          selector: w73 -> [w78 _]
          tunnel: w72 -> [w80 _]
          tunnel: [w74 TRUE] -> w66
          tunnel: w70 -> [w79 _]
          tunnel: w69 -> [w77 _]
          tunnel: w68 -> [w76 _]
          tunnel: w67 -> [w75 _]
          frame No Error {
            n316 = case shown="\"VNA LOOP\", Default" w80 {
              selector: w80 -> [w87 w125 w187 w403 _ w469 w474 w494 w519]
              tunnel: w79 -> [w85 w120 w183 _ _ _ _ _ _]
              tunnel: w78 -> [_ _ _ _ _ _ _ _ _]
              tunnel: w77 -> [w84 w122 w185 w401 _ _ w473 _ w522]
              tunnel: w76 -> [w83 _ _ _ _ _ _ _ _]
              tunnel: w75 -> [w82 w121 w184 w400 _ _ w472 _ w521]
              tunnel: [FALSE FALSE FALSE FALSE FALSE FALSE FALSE FALSE TRUE] -> w74
              frame "VNA LOOP", Default {
                n317 = local write "STATUS"(w87) -> ()
                n318 = stacked-sequence {
                  tunnel: w84 -> [w97 _]
                  tunnel: w83 -> [_ _]
                  tunnel: w82 -> [w96 _]
                  tunnel: w85 -> [_ w116]
                  frame #0 {
                    (unwired) 10 ("kernel size (pts)")
                    n319 = local read "SPECTRUM POST PROCESSING PARAMETERS"() -> (w92:cluster{"N° SMOOTHING POINTS":i32})
                    n320 = local read "RP VNA SETTING"() -> (w110:T1)
                    n321 = Unbundle By Name(w92) -> ("N° SMOOTHING POINTS"=w91:i32)
                    n322 = Unbundle By Name(w110) -> ("Sweep size"=w109:u32)
                    n323 = local read "RAW Freq table"() -> (w105:dbl[])
                    n324 = local read "VNA DATA CLUSTER"() -> (w95:T8)
                    n325 = call "VNARP-CASES.vi"("entrée d'erreur (pas d'erreur)"=w96, "Setting"=u32 0, "Énum"=T11."SWEEP START", "ID de connexion"=w97) -> ("sortie d'erreur"=w106:errorcluster, "ID de connexion en sortie"=w111:refnum<k5>)  [unwired: 3 in]
                    n326 = call "VNARP-Read.vi"("ID de connexion"=w111, "entrée d'erreur (pas d'erreur)"=w106, "SIZE"=w109) -> ("MAGNITUDE 1"=w108:sgl[], "PHASE 1"=w107:dbl[])  [unwired: 9 in, 6 out]
                    n327 = call "VNARP-BOXCAR.vi"("Y IN"=w108, "kernel size (pts)"=w91, "Freq table IN"=w105) -> ("Y OUT"=w89:dbl[], "Freq table OUT"=w104:dbl[])  [unwired: 1 in]
                    n328 = call "VNARP-BOXCAR.vi"("Y IN"=w107, "kernel size (pts)"=w91, "Freq table IN"=w105) -> ("Y OUT"=w88:dbl[], "Freq table OUT"=w93:dbl[])  [unwired: 1 in]
                    n329 = Bundle By Name(cluster=w95, "FREQUENCY TABLE"=w93, "MAGNITUDE TABLE"=w89, "PHASE TABLE"=w88) -> (w94:T8)
                    n330 = Build Cluster Array(w104, w89) -> (w102:cluster{dbl, dbl}[])
                    n331 = Build Cluster Array(w93, w88) -> (w103:cluster{dbl, dbl}[])
                    n332 = local write "VNA DATA CLUSTER"(w94) -> ()
                    n333 = Bundle(w102) -> (w101:cluster{cluster{dbl, dbl}[]})  [unwired: 1 in]
                    n334 = Bundle(w103) -> (w100:cluster{cluster{dbl, dbl}[]})  [unwired: 1 in]
                    n335 = Build Array(w101, w100) -> (w90:cluster{cluster{dbl, dbl}[]}[])
                    n336 = local write "MAGNITUDE/PHASE"(w90) -> ()
                    n337 = property on="MAGNITUDE/PHASE" class="XYGraph (strict)"("Val(Sgnl)"=w90) -> ()  [unwired: 2 in, 2 out]
                  }
                  frame #1 {
                    n338 = local read "LOOP ACT"() -> (w115:bool)
                    n339 = Select(t="VNA LOOP" ("element"), s=w115, f="WAIT" ("element")) -> (s? t:f=w114:string)
                    n340 = Enqueue Element(queue=w116, element=w114) -> ()  [unwired: 2 in, 3 out]
                    n341 = stacked-sequence {
                      frame #0 {
                        n342 = local write "ACQ Indicator"(TRUE ("ACQ Indicator")) -> ()
                      }
                      frame #1 {
                        n343 = Wait (ms)(milliseconds to wait=u32 100 ("attente (ms)")) -> ()  [unwired: 1 out]
                      }
                      frame #2 {
                        n344 = local write "ACQ Indicator"(FALSE ("ACQ Indicator")) -> ()
                      }
                    }
                  }
                }
                n345 = Wait (ms)(milliseconds to wait=u32 10 ("attente (ms)")) -> ()  [unwired: 1 out]
              }
              frame "TRACK OBS" {
                n346 = local write "STATUS"(w125) -> ()
                n347 = stacked-sequence {
                  tunnel: w122 -> [w135 _ _ _]
                  tunnel: w121 -> [w134 _ _ _]
                  tunnel: w120 -> [_ _ _ w182]
                  frame #0 {
                    n348 = local read "SPECTRUM POST PROCESSING PARAMETERS"() -> (w128:cluster{"N° SMOOTHING POINTS":i32})
                    n349 = local read "RP VNA SETTING"() -> (w148:T1)
                    n350 = Unbundle By Name(w128) -> ("N° SMOOTHING POINTS"=w127:i32)
                    n351 = Unbundle By Name(w148) -> ("Sweep size"=w147:u32)
                    n352 = local read "RAW Freq table"() -> (w143:dbl[])
                    n353 = call "VNARP-CASES.vi"("entrée d'erreur (pas d'erreur)"=w134, "Setting"=u32 0, "Énum"=T11."SWEEP START", "ID de connexion"=w135) -> ("sortie d'erreur"=w144:errorcluster, "ID de connexion en sortie"=w149:refnum<k5>)  [unwired: 3 in]
                    n354 = call "VNARP-Read.vi"("ID de connexion"=w149, "entrée d'erreur (pas d'erreur)"=w144, "SIZE"=w147) -> ("MAGNITUDE 1"=w146:sgl[], "PHASE 1"=w145:dbl[])  [unwired: 9 in, 6 out]
                    n355 = call "VNARP-BOXCAR.vi"("Y IN"=w146, "kernel size (pts)"=w127, "Freq table IN"=w143) -> ("Y OUT"=w130:dbl[], "Freq table OUT"=w142:dbl[])  [unwired: 1 in]
                    n356 = call "VNARP-BOXCAR.vi"("Y IN"=w145, "kernel size (pts)"=w127, "Freq table IN"=w143) -> ("Y OUT"=w129:dbl[], "Freq table OUT"=w131:dbl[])  [unwired: 1 in]
                    n357 = local read "VNA DATA CLUSTER"() -> (w133:T8)
                    n358 = Build Cluster Array(w142, w130) -> (w140:cluster{dbl, dbl}[])
                    n359 = Build Cluster Array(w131, w129) -> (w141:cluster{dbl, dbl}[])
                    n360 = Bundle By Name(cluster=w133, "FREQUENCY TABLE"=w131, "MAGNITUDE TABLE"=w130, "PHASE TABLE"=w129) -> (w132:T8)
                    n361 = Bundle(w140) -> (w139:cluster{cluster{dbl, dbl}[]})  [unwired: 1 in]
                    n362 = Bundle(w141) -> (w138:cluster{cluster{dbl, dbl}[]})  [unwired: 1 in]
                    n363 = Build Array(w139, w138) -> (w126:cluster{cluster{dbl, dbl}[]}[])
                    n364 = local write "MAGNITUDE/PHASE"(w126) -> ()
                    n365 = property on="MAGNITUDE/PHASE" class="XYGraph (strict)"("Val(Sgnl)"=w126) -> ()  [unwired: 2 in, 2 out]
                    n366 = local write "VNA DATA CLUSTER"(w132) -> ()
                  }
                  frame #1 {
                    n367 = local read "RP VNA SETTING"() -> (w159:T1)
                    n368 = local read "VNA DATA CLUSTER"() -> (w162:T8)
                    n369 = Unbundle By Name(w159) -> ("Sweep size"=w158:u32)
                    n370 = Max & Min(x=500 ("Fit length"), y=w158) -> (min(x,y)=w156:u32)  [unwired: 1 out]
                    n371 = Unbundle By Name(w162) -> ("FREQUENCY TABLE"=w155:ext[], "MAGNITUDE TABLE"=w154:ext[])
                    n372 = call "VNARP PARABOLA FIT.vi"("Freq Table IN"=w155, "Fit length"=w156, "Y IN"=w154) -> ("Parabol max position"=w161:dbl)  [unwired: 3 out]
                    n373 = feedback #2() -> (w160:dbl[])
                    n374 = Build Array (concatenate)(w160, w161) -> (w152:dbl[])
                    n375 = call "Search Unsorted 1D Array.vim"("element"=0.0, "unsorted 1D array"=w152) -> ("index of element"=w153:i32)  [unwired: 9 in]
                    n376 = Delete From Array(array=w152, index=w153) -> (array with subset deleted=w150:dbl[])  [unwired: 1 in, 1 out]
                    n377 = feedback-in #2(w150) -> ()
                    n378 = local write "track data"(w150) -> ()
                  }
                  frame #2 {
                    n379 = local read "TEMPORAL SMOOTHING"() -> (w165:i32)
                    n380 = local read "track data"() -> (w163:dbl[])
                    n381 = Array Size(array=w163) -> (size(s)=w167:i32)
                    n382 = Subtract(x=w167, y=w165) -> (x-y=w168:i32)
                    n383 = for {
                      N: w168 -> [_]
                      tunnel: w165 -> [w176]
                      tunnel: w163 -> [w177]
                      tunnel: [w173] -> w166 mode=indexing
                      i -> [w175]
                      n384 = Array Subset(array=w177, index=w175, length=w176) -> (w174:dbl[])
                      n385 = call-poly <vilib>:"Mean.vi"("X"=w174) -> ("mean"=w173:dbl)  [unwired: 1 out]
                    }
                    n386 = local read "N°POINTS TO DISPLAY"() -> (w169:i32)
                    n387 = Array Size(array=w166) -> (size(s)=w171:i32)
                    n388 = Subtract(x=w171, y=w169) -> (x-y=w170:i32)
                    n389 = Max & Min(x=0.0, y=w170) -> (max(x,y)=w172:dbl)  [unwired: 1 out]
                    n390 = Array Subset(array=w166, index=w172, length=w169) -> ()  [unwired: 1 out]
                  }
                  frame #3 {
                    n391 = local read "LOOP ACT"() -> (w181:bool)
                    n392 = Select(t="TRACK" ("element"), s=w181, f="WAIT" ("element")) -> (s? t:f=w180:string)
                    n393 = Enqueue Element(queue=w182, element=w180) -> ()  [unwired: 2 in, 3 out]
                  }
                }
                n394 = Wait (ms)(milliseconds to wait=u32 10 ("attente (ms)")) -> ()  [unwired: 1 out]
              }
              frame "TRACK" {
                n395 = local write "STATUS"(w187) -> ()
                n396 = stacked-sequence {
                  tunnel: w185 -> [_ w194 _]
                  tunnel: w184 -> [_ w193 _]
                  tunnel: w183 -> [_ w192 w395]
                  frame #0 {
                    n397 = local read "DELAY BETWEEN TRIG (s)"() -> (w190:i32)
                    n398 = Multiply(x=w190, y=u32 1000 ("attente (ms)")) -> (x*y=w189:u32)
                    n399 = Wait (ms)(milliseconds to wait=w189) -> ()  [unwired: 1 out]
                  }
                  frame #1 {
                    n400 = local read "CHANNELS PARAMETERS"() -> (w191:T4)
                    n401 = for {
                      tunnel: w191 -> [w200] mode=indexing
                      tunnel: w194 -> [w199]
                      tunnel: w193 -> [w198]
                      tunnel: w192 -> [w196]
                      tunnel: w191 -> [w195]
                      i -> [w197]
                      n402 = Unbundle By Name(w200) -> ("CHANNEL TRACK ?"=w201:bool)
                      n403 = case shown="True" w201 {
                        tunnel: w200 -> [_ w203]
                        tunnel: w199 -> [_ w204]
                        tunnel: w198 -> [_ w206]
                        tunnel: w197 -> [_ w205]
                        tunnel: w196 -> [_ _]
                        tunnel: w195 -> [_ w202]
                        frame False {
                        }
                        frame True {
                          n404 = stacked-sequence {
                            tunnel: w206 -> [_ w218 _ _ _ w247 w264 _ _ _ _ _ _ _]
                            tunnel: w205 -> [w207 _ _ _ w238 _ _ w286 w291 w307 _ _ _ _]
                            tunnel: w204 -> [_ w209 _ _ _ w244 w262 _ _ _ _ _ _ _]
                            tunnel: w203 -> [_ w208 _ _ w239 _ _ _ _ _ _ _ _ _]
                            tunnel: w202 -> [_ _ _ _ w237 _ _ _ _ _ _ _ _ _]
                            frame #0 {
                              # "ATTENTION : do not trig channel choice change event !!!!"
                              # "switch"
                              n405 = local write "CHANNEL CHOICE VNA"(w207) -> ()
                              n406 = local write "CHANNELS IND TRACK"(w207) -> ()
                            }
                            frame #1 {
                              n407 = local write "VNA Settings cluster"(w208) -> ()
                              n408 = local read "RP VNA SETTING"() -> (w221:T1)
                              n409 = call "VNARP-VNASETTING CLTR MANAGMENT.vi"("VNA Settings cluster"=w208, "RP VNA SETTING"=w221) -> ("OUTPUT VNA SETTINGS"=w219:T1)  [unwired: 1 in]
                              n410 = local write "RP VNA SETTING"(w219) -> ()
                              n411 = call "VNARP-SettingsUpdate.vi"("Error IN"=w218, "RP VNA SETTINGS IN"=w219, "ID de connexion IN"=w209) -> ("Freq table"=w220:dbl[])  [unwired: 2 out]
                              n412 = local write "RAW Freq table"(w220) -> ()
                              n413 = Unbundle By Name(w208) -> ("START 2"=w211:dbl, "STOP 2"=w217:dbl, "CENTER 2"=w216:dbl, "SPAN 2"=w215:dbl, "PUMP"=w210:dbl, "PROBE"=w214:dbl, "Points N° 2"=w213:i32, "SPACING 2"=w212:dbl)
                              n414 = local write "Points N°"(w213) -> ()
                              n415 = local write "SPACING"(w212) -> ()
                              n416 = local write "CENTER"(w216) -> ()
                              n417 = local write "START"(w211) -> ()
                              n418 = local write "STOP"(w217) -> ()
                              n419 = local write "PROBE"(w214) -> ()
                              n420 = local write "SPAN"(w215) -> ()
                              n421 = local write "PUMP"(w210) -> ()
                              n422 = property on="START" class="DigNum (strict)"("Val(Sgnl)"=w211) -> ()  [unwired: 2 in, 2 out]
                              n423 = property on="PUMP" class="Slide (strict)"("Val(Sgnl)"=w210) -> ()  [unwired: 2 in, 2 out]
                            }
                            frame #2 {
                              w230 = u16 0 items=["AOUT0", "AOUT1", "AOUT2", "AOUT3"] ("Pin #")
                              w229 = u16 1 items=["AOUT0", "AOUT1", "AOUT2", "AOUT3"] ("Pin #")
                              n424 = local read "VOA Calibration cluster"() -> (w228:cluster{"PUMP":dbl[], "PROBE":dbl[]})
                              n425 = local read "NETWORK PARAMETERS"() -> (w232:T7)
                              n426 = Unbundle By Name(w232) -> ("RP-IP 2"=w231:string)
                              n427 = Unbundle By Name(w228) -> ("PUMP"=w223:dbl[], "PROBE"=w226:dbl[])
                              n428 = local read "PUMP"() -> (w224:dbl)
                              n429 = local read "PROBE"() -> (w227:dbl)
                              n430 = call "RP-VOA CONVERSION P to V.vi"("Calibration points"=w223, "% power"=w224) -> ("DAC Voltage"=w222:dbl)
                              n431 = call "RP-VOA CONVERSION P to V.vi"("Calibration points"=w226, "% power"=w227) -> ("DAC Voltage"=w225:dbl)
                              n432 = call "RP-ANALOG-OUT.vi"("Voltage"=w222, "Pin #"=w230, "IP address"=w231) -> ()  [unwired: 1 out]
                              n433 = call "RP-ANALOG-OUT.vi"("Voltage"=w225, "Pin #"=w229, "IP address"=w231) -> ()  [unwired: 1 out]
                            }
                            frame #3 {
                              n434 = local read "VNA Settings cluster"() -> (w236:T10)
                              n435 = local read "PROBE"() -> (w234:dbl)
                              n436 = local read "PUMP"() -> (w235:dbl)
                              n437 = Bundle By Name(cluster=w236, "PUMP"=w235, "PROBE"=w234) -> (w233:T10)
                              n438 = local write "VNA Settings cluster"(w233) -> ()
                            }
                            frame #4 {
                              n439 = local read "VNA Settings cluster"() -> (w242:T10)
                              n440 = Unbundle By Name(w239) -> ("CHANNEL TRACK ?"=w241:bool)
                              n441 = Bundle By Name(cluster=w242, "CHANNEL TRACK ?"=w241) -> (w240:T10)
                              n442 = Replace Array Subset(array=w237, new element=w240, index=w238) -> (w243:T4)
                              n443 = local write "CHANNELS PARAMETERS"(w243) -> ()
                            }
                            frame #5 {
                              # "wait for stab"
                              n444 = local read "DELAY AFTER SWITCH (s)"() -> (w246:i32)
                              n445 = Equal To 0?(x=w246) -> (x = 0?=w245:bool)
                              n446 = case shown="False" w245 {
                                tunnel: w247 -> [w249 _]
                                tunnel: w244 -> [w248 _]
                                frame False {
                                n447 = Tick Count (ms)() -> (millisecond timer value=w250:u32)
                                n448 = while {
                                tunnel: w250 -> [w259]
                                tunnel: w249 -> [w253]
                                tunnel: w248 -> [w252]
                                stop <- w254 stop-if-true
                                n449 = flat-sequence {
                                tunnel: w253 -> [_]
                                tunnel: w252 -> [_]
                                tunnel: [w260] -> w251
                                frame #0 {
                                }
                                frame #1 {
                                n450 = Tick Count (ms)() -> (millisecond timer value=w260:u32)
                                }
                                }
                                n451 = local read "DELAY AFTER SWITCH (s)"() -> (w258:i32)
                                n452 = Subtract(x=w251, y=w259) -> (x-y=w256:u32)
                                n453 = Multiply(x=w258, y=1000) -> (x*y=w255:i32)
                                n454 = Greater Or Equal?(x=w256, y=w255) -> (x >= y?=w254:bool)
                                }
                                }
                                frame True {
                                }
                              }
                            }
                            frame #6 {
                              # "AVERAGING IS MISSING !"
                              n455 = local read "SPECTRUM POST PROCESSING PARAMETERS"() -> (w268:cluster{"N° SMOOTHING POINTS":i32})
                              n456 = Unbundle By Name(w268) -> ("N° SMOOTHING POINTS"=w267:i32)
                              n457 = local read "RP VNA SETTING"() -> (w284:T1)
                              n458 = Unbundle By Name(w284) -> ("Sweep size"=w283:u32)
                              n459 = local read "RAW Freq table"() -> (w279:dbl[])
                              n460 = call "VNARP-CASES.vi"("entrée d'erreur (pas d'erreur)"=w264, "Setting"=u32 0, "Énum"=T11."SWEEP START", "ID de connexion"=w262) -> ("sortie d'erreur"=w280:errorcluster, "ID de connexion en sortie"=w285:refnum<k5>)  [unwired: 3 in]
                              n461 = local read "CHANNEL CHOICE VNA"() -> (w263:T3)
                              n462 = call "VNARP-Read.vi"("ID de connexion"=w285, "entrée d'erreur (pas d'erreur)"=w280, "SIZE"=w283) -> ("MAGNITUDE 1"=w282:sgl[], "PHASE 1"=w281:dbl[])  [unwired: 9 in, 6 out]
                              n463 = call "VNARP-BOXCAR.vi"("Y IN"=w282, "kernel size (pts)"=w267, "Freq table IN"=w279) -> ("Y OUT"=w270:dbl[], "Freq table OUT"=w278:dbl[])  [unwired: 1 in]
                              n464 = call "VNARP-BOXCAR.vi"("Y IN"=w281, "kernel size (pts)"=w267, "Freq table IN"=w279) -> ("Y OUT"=w269:dbl[], "Freq table OUT"=w271:dbl[])  [unwired: 1 in]
                              n465 = Build Cluster Array(w278, w270) -> (w276:cluster{dbl, dbl}[])
                              n466 = Build Cluster Array(w271, w269) -> (w277:cluster{dbl, dbl}[])
                              n467 = local read "VNA DATA CLUSTER"() -> (w273:T8)
                              n468 = Bundle By Name(cluster=w273, "CHANNEL"=w263, "FREQUENCY TABLE"=w271, "MAGNITUDE TABLE"=w270, "PHASE TABLE"=w269) -> (w272:T8)
                              n469 = Bundle(w276) -> (w275:cluster{cluster{dbl, dbl}[]})  [unwired: 1 in]
                              n470 = Bundle(w277) -> (w274:cluster{cluster{dbl, dbl}[]})  [unwired: 1 in]
                              n471 = Build Array(w275, w274) -> (w261:cluster{cluster{dbl, dbl}[]}[])
                              n472 = local write "MAGNITUDE/PHASE"(w261) -> ()
                              n473 = property on="MAGNITUDE/PHASE" class="XYGraph (strict)"("Val(Sgnl)"=w261) -> ()  [unwired: 2 in, 2 out]
                              n474 = local write "VNA DATA CLUSTER"(w272) -> ()
                            }
                            frame #7 {
                              n475 = local read "VNA DATA CLUSTER TBL"() -> (w288:T9)
                              n476 = local read "VNA DATA CLUSTER"() -> (w287:T8)
                              n477 = Replace Array Subset(array=w288, new element=w287, index=w286) -> (w289:T9)
                              n478 = local write "VNA DATA CLUSTER TBL"(w289) -> ()
                            }
                            frame #8 {
                              n479 = local read "BTN AUTOSAVE RAW DATA"() -> (w290:bool)
                              n480 = case shown="True" w290 {
                                tunnel: w291 -> [_ w293]
                                frame False {
                                }
                                frame True {
                                # "save to file vna"
                                n481 = local read "VNA DATA CLUSTER TBL"() -> (w304:T9)
                                n482 = local read "Track Repositery List"() -> (w294:path[])
                                n483 = Tick Count (ms)() -> (millisecond timer value=w302:u32)
                                n484 = Number To Decimal String(number=w302) -> (decimal integer string=w301:string)  [unwired: 1 in]
                                n485 = call "RP-VNA DATA TBL Extract.vi"("VNA DATA CLUSTER TBL"=w304, "index"=w293) -> ("appended array"=w303:ext[][])  [unwired: 2 in, 1 out]
                                n486 = Concatenate Strings("RAW VNA DATA " ("string"), w301, ".txt" ("string")) -> (w299:string)
                                n487 = Index Array(array=w294, index=w293) -> (element=w292:path)
                                n488 = Build Path(base path=w292, name or relative path=w299) -> (appended path=w298:path)
                                n489 = call-poly <vilib>:"Write Delimited Spreadsheet.vi"("file path (dialog if empty)"=w298, "format (%.3f)"="%.6f", "2D data"=w303, "transpose? (no:F)"=TRUE) -> ()  [unwired: 10 in, 2 out]
                                }
                              }
                            }
                            frame #9 {
                              # "add to track kpi tables"
                              n490 = local read "TRACK DATA CLUSTER TBL"() -> (w308:cluster{"CHANNEL":dbl, "KPI 1 TRACK":ext[]}[])
                              n491 = local read "VNA DATA CLUSTER"() -> (w319:T8)
                              n492 = local read "RP VNA SETTING"() -> (w318:T1)
                              n493 = Unbundle By Name(w318) -> ("Sweep size"=w317:u32)
                              n494 = Unbundle By Name(w319) -> ("FREQUENCY TABLE"=w315:ext[], "MAGNITUDE TABLE"=w314:ext[])
                              n495 = Index Array(array=w308, index=w307) -> (element=w310:cluster{"CHANNEL":dbl, "KPI 1 TRACK":ext[]})
                              n496 = Unbundle By Name(w310) -> ("KPI 1 TRACK"=w312:ext[])
                              n497 = Max & Min(x=500 ("Fit length"), y=w317) -> (min(x,y)=w316:u32)  [unwired: 1 out]
                              n498 = call "VNARP PARABOLA FIT.vi"("Freq Table IN"=w315, "Fit length"=w316, "Y IN"=w314) -> ("Parabol max position"=w305:dbl)  [unwired: 3 out]
                              n499 = Build Array (concatenate)(w312, w305) -> (w311:ext[])
                              n500 = Bundle By Name(cluster=w310, "CHANNEL"=w307, "KPI 1 TRACK"=w311) -> (w309:cluster{"CHANNEL":dbl, "KPI 1 TRACK":ext[]})
                              n501 = Replace Array Subset(array=w308, new element=w309, index=w307) -> (w306:cluster{"CHANNEL":dbl, "KPI 1 TRACK":ext[]}[])
                              n502 = local write "TRACK DATA CLUSTER TBL"(w306) -> ()
                            }
                            frame #10 {
                              n503 = local read "TRACK DATA CLUSTER TBL"() -> (w323:cluster{"CHANNEL":dbl, "KPI 1 TRACK":ext[]}[])
                              n504 = for {
                                tunnel: w323 -> [w348] mode=indexing
                                tunnel: [w326] -> w322 mode=indexing
                                tunnel: [w325] -> w321 mode=indexing
                                tunnel: [w324] -> w320 mode=indexing
                                n505 = local read "TEMPORAL SMOOTHING"() -> (w345:i32)
                                n506 = Unbundle By Name(w348) -> ("KPI 1 TRACK"=w344:ext[])
                                n507 = Array Size(array=w344) -> (size(s)=w346:i32)
                                n508 = Subtract(x=w346, y=w345) -> (x-y=w347:i32)
                                n509 = for {
                                N: w347 -> [_]
                                tunnel: w345 -> [w352]
                                tunnel: w344 -> [w353]
                                tunnel: [w349] -> w333 mode=indexing
                                i -> [w351]
                                n510 = Array Subset(array=w353, index=w351, length=w352) -> (w350:ext[])
                                n511 = call-poly <vilib>:"Mean.vi"("X"=w350) -> ("mean"=w349:dbl)  [unwired: 1 out]
                                }
                                n512 = Delete From Array(array=w333, length=1, index=0) -> (array with subset deleted=w325:dbl[])  [unwired: 1 out]
                                n513 = local read "DISPLAY OPTION"() -> (w342:u16)
                                n514 = Index Array(array=w325, index=0) -> (element=w337:dbl)
                                n515 = local read "N°POINTS TO DISPLAY"() -> (w329:i32)
                                n516 = Subtract(x=w325, y=w337) -> (x-y=w338:dbl[])
                                n517 = Divide(x=w338, y=w337) -> (x/y=w336:dbl[])
                                n518 = Equal?(x=w342, y=u16 0) -> (x = y?=w334:bool)
                                n519 = Multiply(x=w336, y=1000000.0 ("f")) -> (x*y=w324:dbl[])
                                n520 = Select(t=w325, s=w334, f=w324) -> (s? t:f=w327:dbl[])
                                n521 = Array Size(array=w327) -> (size(s)=w331:i32)
                                n522 = Subtract(x=w331, y=w329) -> (x-y=w330:i32)
                                n523 = Max & Min(x=0.0, y=w330) -> (max(x,y)=w332:dbl)  [unwired: 1 out]
                                n524 = Array Subset(array=w327, index=w332) -> (w326:dbl[])  [unwired: 1 in]
                              }
                              n525 = local write "TRACK DATA ABS"(w321) -> ()
                              n526 = local write "TRACK DATA REL"(w320) -> ()
                              n527 = local write "LIVE TRACK"(w322) -> ()
                            }
                            frame #11 {
                              n528 = local read "TRACK DATA CLUSTER TBL"() -> (w356:cluster{"CHANNEL":dbl, "KPI 1 TRACK":ext[]}[])
                              n529 = for {
                                tunnel: w356 -> [w369] mode=indexing
                                tunnel: [w360] -> w355 mode=indexing
                                tunnel: [w359] -> w354 mode=indexing
                                n530 = Unbundle By Name(w369) -> ("KPI 1 TRACK"=w358:ext[])
                                n531 = local read "DISPLAY OPTION"() -> (w367:u16)
                                n532 = Delete From Array(array=w358, length=1, index=0) -> (array with subset deleted=w360:ext[])  [unwired: 1 out]
                                n533 = Equal?(x=w367, y=u16 0) -> ()  [unwired: 1 out]
                                n534 = Index Array(array=w360, index=0) -> (element=w362:ext)
                                n535 = Subtract(x=w360, y=w362) -> (x-y=w363:ext[])
                                n536 = Divide(x=w363, y=w362) -> (x/y=w361:ext[])
                                n537 = Multiply(x=w361, y=1000000.0 ("f")) -> (x*y=w359:ext[])
                              }
                              n538 = local write "TRACK DATA ABS NO SMOOTHING"(w355) -> ()
                              n539 = local write "TRACK DATA REL NO SMOOTHING"(w354) -> ()
                            }
                            frame #12 {
                              n540 = local read "TRACK DATA ABS NO SMOOTHING"() -> (w378:dbl[][])
                              n541 = local read "TRACK REPOSITERY"() -> (w391:path)
                              n542 = local read "TRACK REPOSITERY"() -> (w372:path)
                              n543 = local read "TRACK DATA ABS"() -> (w385:dbl[][])
                              n544 = Build Path(base path=w391, name or relative path="ALL CHANNEL ABS Track.txt") -> (appended path=w392:path)
                              n545 = Build Path(base path=w372, name or relative path="ALL CHANNEL ABS Track NS.txt") -> (appended path=w371:path)
                              n546 = call-poly <vilib>:"Write Delimited Spreadsheet.vi"("file path (dialog if empty)"=w392, "format (%.3f)"="%.6f", "2D data"=w385, "transpose? (no:F)"=TRUE) -> ()  [unwired: 10 in, 2 out]
                              n547 = call-poly <vilib>:"Write Delimited Spreadsheet.vi"("file path (dialog if empty)"=w371, "format (%.3f)"="%.6f", "2D data"=w378, "transpose? (no:F)"=TRUE) -> ()  [unwired: 10 in, 2 out]
                              n548 = local read "TRACK DATA REL NO SMOOTHING"() -> (w379:dbl[][])
                              n549 = local read "TRACK REPOSITERY"() -> (w388:path)
                              n550 = local read "TRACK REPOSITERY"() -> (w375:path)
                              n551 = local read "TRACK DATA REL"() -> (w384:dbl[][])
                              n552 = Build Path(base path=w388, name or relative path="ALL CHANNEL REL Track.txt") -> (appended path=w387:path)
                              n553 = Build Path(base path=w375, name or relative path="ALL CHANNEL REL Track NS.txt") -> (appended path=w376:path)
                              n554 = call-poly <vilib>:"Write Delimited Spreadsheet.vi"("file path (dialog if empty)"=w387, "format (%.3f)"="%.6f", "2D data"=w384, "transpose? (no:F)"=TRUE) -> ()  [unwired: 10 in, 2 out]
                              n555 = call-poly <vilib>:"Write Delimited Spreadsheet.vi"("file path (dialog if empty)"=w376, "format (%.3f)"="%.6f", "2D data"=w379, "transpose? (no:F)"=TRUE) -> ()  [unwired: 10 in, 2 out]
                            }
                            frame #13 {
                            }
                          }
                        }
                      }
                    }
                  }
                  frame #2 {
                    n556 = local read "LOOP ACT"() -> (w398:bool)
                    n557 = Select(t="TRACK" ("element"), s=w398, f="WAIT" ("element")) -> (s? t:f=w397:string)
                    n558 = Enqueue Element(queue=w395, element=w397) -> ()  [unwired: 2 in, 3 out]
                  }
                }
              }
              frame "RUN VNA" {
                n559 = local write "STATUS"(w403) -> ()
                n560 = stacked-sequence {
                  tunnel: w401 -> [w427 _]
                  tunnel: w400 -> [w426 _]
                  frame #0 {
                    n561 = local read "RP VNA SETTING"() -> (w422:T1)
                    n562 = local read "SPECTRUM POST PROCESSING PARAMETERS"() -> (w407:cluster{"N° SMOOTHING POINTS":i32})
                    n563 = Unbundle By Name(w407) -> ("N° SMOOTHING POINTS"=w405:i32)
                    n564 = Unbundle By Name(w422) -> ("Sweep size"=w421:u32)
                    n565 = local read "RAW Freq table"() -> (w417:dbl[])
                    n566 = call "VNARP-CASES.vi"("entrée d'erreur (pas d'erreur)"=w426, "Setting"=u32 0, "Énum"=T11."SWEEP START", "ID de connexion"=w427) -> ("sortie d'erreur"=w418:errorcluster, "ID de connexion en sortie"=w423:refnum<k5>)  [unwired: 3 in]
                    n567 = local read "VNA DATA CLUSTER"() -> (w411:T8)
                    n568 = call "VNARP-Read.vi"("ID de connexion"=w423, "entrée d'erreur (pas d'erreur)"=w418, "SIZE"=w421) -> ("MAGNITUDE 1"=w420:sgl[], "PHASE 1"=w419:dbl[])  [unwired: 9 in, 6 out]
                    n569 = call "VNARP-BOXCAR.vi"("Y IN"=w420, "kernel size (pts)"=w405, "Freq table IN"=w417) -> ("Y OUT"=w406:dbl[], "Freq table OUT"=w409:dbl[])  [unwired: 1 in]
                    n570 = call "VNARP-BOXCAR.vi"("Y IN"=w419, "kernel size (pts)"=w405, "Freq table IN"=w417) -> ("Y OUT"=w408:dbl[], "Freq table OUT"=w416:dbl[])  [unwired: 1 in]
                    n571 = Bundle By Name(cluster=w411, "FREQUENCY TABLE"=w409, "MAGNITUDE TABLE"=w406, "PHASE TABLE"=w408) -> (w410:T8)
                    n572 = Build Cluster Array(w409, w406) -> (w414:cluster{dbl, dbl}[])
                    n573 = Build Cluster Array(w416, w408) -> (w415:cluster{dbl, dbl}[])
                    n574 = local write "VNA DATA CLUSTER"(w410) -> ()
                    n575 = Bundle(w414) -> (w413:cluster{cluster{dbl, dbl}[]})  [unwired: 1 in]
                    n576 = Bundle(w415) -> (w412:cluster{cluster{dbl, dbl}[]})  [unwired: 1 in]
                    n577 = Build Array(w413, w412) -> (w404:cluster{cluster{dbl, dbl}[]}[])
                    n578 = local write "MAGNITUDE/PHASE"(w404) -> ()
                    n579 = property on="MAGNITUDE/PHASE" class="XYGraph (strict)"("Val(Sgnl)"=w404) -> ()  [unwired: 2 in, 2 out]
                  }
                  frame #1 {
                    n580 = stacked-sequence {
                      frame #0 {
                        n581 = local write "ACQ Indicator"(TRUE ("ACQ Indicator")) -> ()
                      }
                      frame #1 {
                        n582 = Wait (ms)(milliseconds to wait=u32 100 ("attente (ms)")) -> ()  [unwired: 1 out]
                      }
                      frame #2 {
                        n583 = local write "ACQ Indicator"(FALSE ("ACQ Indicator")) -> ()
                      }
                    }
                  }
                }
                n584 = Wait (ms)(milliseconds to wait=u32 10 ("attente (ms)")) -> ()  [unwired: 1 out]
              }
              frame "CHANNEL CHANGE" {
                n585 = stacked-sequence {
                  frame #0 {
                    n586 = local read "CHANNEL CHOICE VNA"() -> (w443:T3)
                    n587 = local read "CHANNELS PARAMETERS"() -> (w444:T4)
                    n588 = Index Array(array=w444, index=w443) -> (element=w440:T10)
                    n589 = local write "VNA Settings cluster"(w440) -> ()
                    n590 = local read "RP VNA SETTING"() -> (w441:T1)
                    n591 = Unbundle By Name(w440) -> ("START 2"=w434:dbl, "STOP 2"=w439:dbl, "CENTER 2"=w438:dbl, "SPAN 2"=w437:dbl, "PUMP"=w432:dbl, "PROBE"=w433:dbl, "Points N° 2"=w436:i32, "SPACING 2"=w435:dbl)
                    n592 = local write "Points N°"(w436) -> ()
                    n593 = local write "SPACING"(w435) -> ()
                    n594 = local write "CENTER"(w438) -> ()
                    n595 = local write "START"(w434) -> ()
                    n596 = local write "STOP"(w439) -> ()
                    n597 = local write "PROBE"(w433) -> ()
                    n598 = local write "SPAN"(w437) -> ()
                    n599 = local write "PUMP"(w432) -> ()
                    n600 = call "VNARP-VNASETTING CLTR MANAGMENT.vi"("VNA Settings cluster"=w440, "RP VNA SETTING"=w441) -> ("OUTPUT VNA SETTINGS"=w442:T1)  [unwired: 1 in]
                    n601 = local write "RP VNA SETTING"(w442) -> ()
                    n602 = property on="START" class="DigNum (strict)"("Val(Sgnl)"=w434) -> ()  [unwired: 2 in, 2 out]
                  }
                  frame #1 {
                    w455 = u16 0 items=["AOUT0", "AOUT1", "AOUT2", "AOUT3"] ("Pin #")
                    w454 = u16 1 items=["AOUT0", "AOUT1", "AOUT2", "AOUT3"] ("Pin #")
                    n603 = local read "VOA Calibration cluster"() -> (w453:cluster{"PUMP":dbl[], "PROBE":dbl[]})
                    n604 = local read "NETWORK PARAMETERS"() -> (w456:T7)
                    n605 = local read "PROBE"() -> (w452:dbl)
                    n606 = Unbundle By Name(w456) -> ("RP-IP 2"=w446:string)
                    n607 = Unbundle By Name(w453) -> ("PUMP"=w447:dbl[], "PROBE"=w451:dbl[])
                    n608 = local read "PUMP"() -> (w448:dbl)
                    n609 = local read "CHANNEL CHOICE VNA"() -> (w445:T3)
                    n610 = call "RP-VOA CONVERSION P to V.vi"("Calibration points"=w447, "% power"=w448) -> ("DAC Voltage"=w449:dbl)
                    n611 = call "RP-VOA CONVERSION P to V.vi"("Calibration points"=w451, "% power"=w452) -> ("DAC Voltage"=w450:dbl)
                    n612 = call "RP-ANALOG-OUT.vi"("Voltage"=w449, "Pin #"=w455, "IP address"=w446) -> ()  [unwired: 1 out]
                    n613 = call "RP-ANALOG-OUT.vi"("Voltage"=w450, "Pin #"=w454, "IP address"=w446) -> ()  [unwired: 1 out]
                    n614 = call "RP-SWITCH CHANNEL.vi"("Channel"=w445, "IP address"=w446) -> ()  [unwired: 1 in, 1 out]
                  }
                  frame #2 {
                    n615 = local read "VNA Settings cluster"() -> (w460:T10)
                    n616 = local read "PROBE"() -> (w458:dbl)
                    n617 = local read "PUMP"() -> (w459:dbl)
                    n618 = Bundle By Name(cluster=w460, "PUMP"=w459, "PROBE"=w458) -> (w457:T10)
                    n619 = local write "VNA Settings cluster"(w457) -> ()
                  }
                  frame #3 {
                    n620 = local read "CHANNELS PARAMETERS"() -> (w466:T4)
                    n621 = local read "CHANNEL CHOICE VNA"() -> (w465:T3)
                    n622 = Index Array(array=w466, index=w465) -> (element=w464:T10)
                    n623 = local read "VNA Settings cluster"() -> (w463:T10)
                    n624 = Unbundle By Name(w464) -> ("CHANNEL TRACK ?"=w462:bool)
                    n625 = Bundle By Name(cluster=w463, "CHANNEL TRACK ?"=w462) -> (w461:T10)
                    n626 = Replace Array Subset(array=w466, new element=w461, index=w465) -> (w467:T4)
                    n627 = local write "CHANNELS PARAMETERS"(w467) -> ()
                  }
                  frame #4 {
                    n628 = local read "CHANNEL CHOICE VNA"() -> (→"CHANNEL CHOSEN":T3)
                  }
                }
              }
              frame "WAIT" {
                n629 = local write "STATUS"(w469) -> ()
              }
              frame "UPDATE" {
                n630 = local write "STATUS"(w474) -> ()
                n631 = stacked-sequence {
                  tunnel: w473 -> [w478 _ _]
                  tunnel: w472 -> [w476 _ _]
                  frame #0 {
                    n632 = local read "RP VNA SETTING"() -> (w477:T1)
                    n633 = call "VNARP-SettingsUpdate.vi"("Error IN"=w476, "RP VNA SETTINGS IN"=w477, "ID de connexion IN"=w478) -> ("Freq table"=w475:dbl[])  [unwired: 2 out]
                    n634 = local write "RAW Freq table"(w475) -> ()
                  }
                  frame #1 {
                    n635 = local read "VNA Settings cluster"() -> (w486:T10)
                    n636 = local read "Points N°"() -> (w480:i32)
                    n637 = local read "SPACING"() -> (w479:dbl)
                    n638 = local read "CENTER"() -> (w482:dbl)
                    n639 = local read "START"() -> (w485:dbl)
                    n640 = local read "SPAN"() -> (w481:dbl)
                    n641 = local read "STOP"() -> (w484:dbl)
                    n642 = Bundle By Name(cluster=w486, "START 2"=w485, "STOP 2"=w484, "CENTER 2"=w482, "SPAN 2"=w481, "Points N° 2"=w480, "SPACING 2"=w479) -> (w483:T10)
                    n643 = local write "VNA Settings cluster"(w483) -> ()
                  }
                  frame #2 {
                    n644 = local read "CHANNELS PARAMETERS"() -> (w492:T4)
                    n645 = local read "CHANNEL CHOICE VNA"() -> (w491:T3)
                    n646 = Index Array(array=w492, index=w491) -> (element=w490:T10)
                    n647 = local read "VNA Settings cluster"() -> (w489:T10)
                    n648 = Unbundle By Name(w490) -> ("CHANNEL TRACK ?"=w488:bool)
                    n649 = Bundle By Name(cluster=w489, "CHANNEL TRACK ?"=w488) -> (w487:T10)
                    n650 = Replace Array Subset(array=w492, new element=w487, index=w491) -> (w493:T4)
                    n651 = local write "CHANNELS PARAMETERS"(w493) -> ()
                  }
                }
              }
              frame "POWER UPDATE" {
                n652 = local write "STATUS"(w494) -> ()
                n653 = stacked-sequence {
                  frame #0 {
                    w504 = u16 0 items=["AOUT0", "AOUT1", "AOUT2", "AOUT3"] ("Pin #")
                    w506 = u16 1 items=["AOUT0", "AOUT1", "AOUT2", "AOUT3"] ("Pin #")
                    n654 = local read "VOA Calibration cluster"() -> (w502:cluster{"PUMP":dbl[], "PROBE":dbl[]})
                    n655 = local read "NETWORK PARAMETERS"() -> (w505:T7)
                    n656 = Unbundle By Name(w505) -> ("RP-IP 2"=w503:string)
                    n657 = Unbundle By Name(w502) -> ("PUMP"=w497:dbl[], "PROBE"=w500:dbl[])
                    n658 = local read "PUMP"() -> (w498:dbl)
                    n659 = local read "PROBE"() -> (w501:dbl)
                    n660 = call "RP-VOA CONVERSION P to V.vi"("Calibration points"=w497, "% power"=w498) -> ("DAC Voltage"=w496:dbl)
                    n661 = call "RP-VOA CONVERSION P to V.vi"("Calibration points"=w500, "% power"=w501) -> ("DAC Voltage"=w499:dbl)
                    n662 = call "RP-ANALOG-OUT.vi"("Voltage"=w499, "Pin #"=w506, "IP address"=w503) -> ()  [unwired: 1 out]
                    n663 = call "RP-ANALOG-OUT.vi"("Voltage"=w496, "Pin #"=w504, "IP address"=w503) -> ()  [unwired: 1 out]
                  }
                  frame #1 {
                    n664 = local read "VNA Settings cluster"() -> (w510:T10)
                    n665 = local read "PROBE"() -> (w508:dbl)
                    n666 = local read "PUMP"() -> (w509:dbl)
                    n667 = Bundle By Name(cluster=w510, "PUMP"=w509, "PROBE"=w508) -> (w507:T10)
                    n668 = local write "VNA Settings cluster"(w507) -> ()
                  }
                  frame #2 {
                    n669 = local read "CHANNELS PARAMETERS"() -> (w516:T4)
                    n670 = local read "CHANNEL CHOICE VNA"() -> (w515:T3)
                    n671 = Index Array(array=w516, index=w515) -> (element=w514:T10)
                    n672 = local read "VNA Settings cluster"() -> (w513:T10)
                    n673 = Unbundle By Name(w514) -> ("CHANNEL TRACK ?"=w512:bool)
                    n674 = Bundle By Name(cluster=w513, "CHANNEL TRACK ?"=w512) -> (w511:T10)
                    n675 = Replace Array Subset(array=w516, new element=w511, index=w515) -> (w517:T4)
                    n676 = local write "CHANNELS PARAMETERS"(w517) -> ()
                  }
                }
              }
              frame "STOP" {
                w520 = FALSE ("TRACK-STOP")
                n677 = local write "STATUS"(w519) -> ()
                n678 = local read "RP CONNECT"() -> (w518:bool)
                n679 = case shown="True" w518 {
                  tunnel: w522 -> [_ w525]
                  tunnel: w521 -> [_ w524]
                  frame False {
                  }
                  frame True {
                    n680 = TCP Close Connection(connection ID=w525, error in (no error)=w524) -> ()  [unwired: 1 in, 2 out]
                  }
                }
                n681 = local write "TRACK-STOP"(w520) -> ()
                n682 = local write "LOOP ACT"(w520) -> ()
              }
            }
          }
          frame Error {
          }
        }
      }
      n683 = And(x=w52, y=w51) -> (x .and. y?=w50:bool)
      n684 = case shown="True" w50 {
        tunnel: w61 -> [_ w65]
        tunnel: w59 -> [_ w64]
        frame False {
        }
        frame True {
          n685 = Release Queue(queue=w64, error in (no error)=w65) -> ()  [unwired: 1 in, 3 out]
          n686 = property on="MAIN TAB" class="TabCtl (strict)"("Tabs Visible?"=TRUE ("Onglets visibles ?")) -> ()  [unwired: 2 in, 2 out]
        }
      }
    }
  }
